vi "Live Capture Functional Stack.12.64bit.vi"() -> ()   [LabVIEW 2014]
uses:
  subvis/Stack Track.ctl
  subvis/Stack_State.ctl
  CameraControlTypeDef.ctl
  Desktop/camtiff/ctiff.llb/__CTIFFNewFileAndStyleUINT16.vi
  Desktop/camtiff/ctiff.llb/__CTIFFAddNewPageUINT16.vi
panel:
  out "Stacks":i32
  in  "ROI":bool
  out "Video":T1(plugin-control)
  out "Internal Line Interval":dbl
  in  "Mode":bool
  in  "Preview":bool
  in  "Capture Mode":bool
  out "Record Ready":bool
  in  "Stacks":dbl=1.0
  out "Stack Frames":i32=100
  in  "Stack Frames":i32=100
  in  "Temp":path=path "C:/temp.tmp"
  in  "Frames":i32=100
  in  "HardDisk Record":bool
  in  "Internal Line Interval":dbl
  in  "Slit Width / Lines":sgl=150.0
  in  "Camera Readout Mode":u16(ring)=12 items=["Full Frame"=1, "Slit Scanning"=12]
  in  "Readout Direction":sgl(ring)=1.0 items=["Forward"=1, "Backward"=2]
  in  "Trigger Mode":sgl(ring)=1.0 items=["Normal"=1, "Start "=6]
  in  "Trigger Source":sgl(ring)=2.0 items=["Internal"=1, "External"=2]
  out "State":T2=enum."Start Sequence"
  out "Saving":bool
  in  "AutoIncrement":bool=TRUE
  in  "Path":path=path "C:/Users/spim/Desktop/Craig Cap/temp/a.tiff"
  in  "Frames":i32=100
  out "Frame Index":i32
  out "error out":errorcluster
  in  "stop":bool
  in  "Ram Record":bool
  out "Total Frames":i32
  out "Elapsed Time":u32
  out "Software FPS":dbl
  out "Camera FPS":dbl
  in  "H Offset":i32 min=0 max=0 step=4
  in  "H Width":i32 min=4 max=2048 step=4
  out "SMD":dbl
  out "SHO":i32
  in  "V Offset":i32 min=0 max=0 step=4
  in  "V Width":i32 min=4 max=2048 step=4
  in  "Binning":u16(ring) items=["1x1"=1, "2x2"=2, "4x4"=4]
  out "SHW":i32
  out "SVO":i32
  out "SVW":i32
  in  "Scan Mode":dbl min=1.0 max=2.0 step=1.0
  in  "Exposure":dbl min=0.0010036691729323308 max=10.000004210526315 step=1e-08
  out "EXP":dbl
  out "Camera Model":string
  out "Camera Version":string
  out "Camera Serial":string
  # "Broked"
  # "XYT \nXYZ\nXYTZ\nXYZT"
  # "Capture Mode"
  # "Preview Mode"
  # "HDD superior, will not drop frames or stacks"
  # "Change to rock switch"
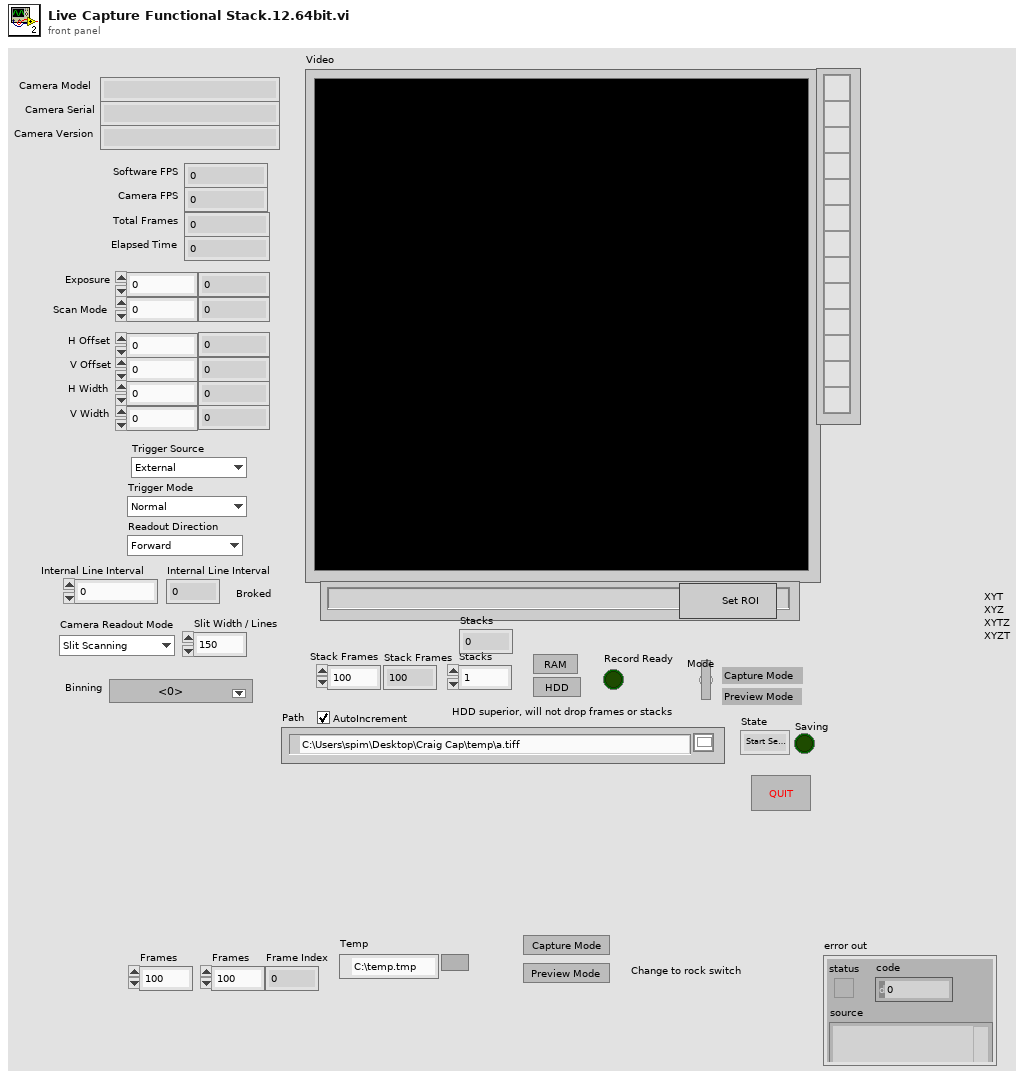
[diagram p1: front panel]
types:
  T1 = typedef "IMAQ Image.ctl" = refnum<image>
  T2 = typedef "Stack Track.ctl" = enum16{"Idle", "Start Sequence", "Read Disk", "STOP", "Collecting", "End"}
  T3 = typedef "CameraControlTypeDef.ctl" = enum16{"IntervalLineInt", "Ram Record", "HardDisk Record", "Disengage Update", "Update", "Idle", "ROI", "Binning", "Scan Mode", "Trigger Mode", "Readout Mode", "Readout Direction", "Preview", "ROIWindow", "Trigger Source"}
  T4 = typedef "Stack_State.ctl" = cluster{"State":T2, "Stack Number":i32, "Image":u16[][], "Stacks":i32}
  T5 = enum8{"Enabled", "Disabled", "Disabled and Grayed Out"}
  T6 = typedef "Image Type" = u32
  T7 = cluster{"Model":string, "Camera ID":string, "Firmware":string}
  T8 = cluster{"Value":i32, "Minimum":i32, "Maximum":i32, "Increment":i32}
  T9 = cluster{"height":u32, "width":u32, "datatype":u32}
  T10 = cluster{"H Offset":i32, "V Offset":i32, "H Width":i32, "V Width":i32}
  T11 = typedef "ROI Descriptor" = cluster{"Global Rectangle":i32[], "Contours":cluster{"ID":enum32{"External", "Internal"}, "Type":u32, "Coordinates":i32[]}[]}
  T12 = cluster{"ID":enum32{"External", "Internal"}, "Type":u32, "Coordinates":i32[]}[]
  T13 = cluster{"ID":enum32{"External", "Internal"}, "Type":u32, "Coordinates":i32[]}
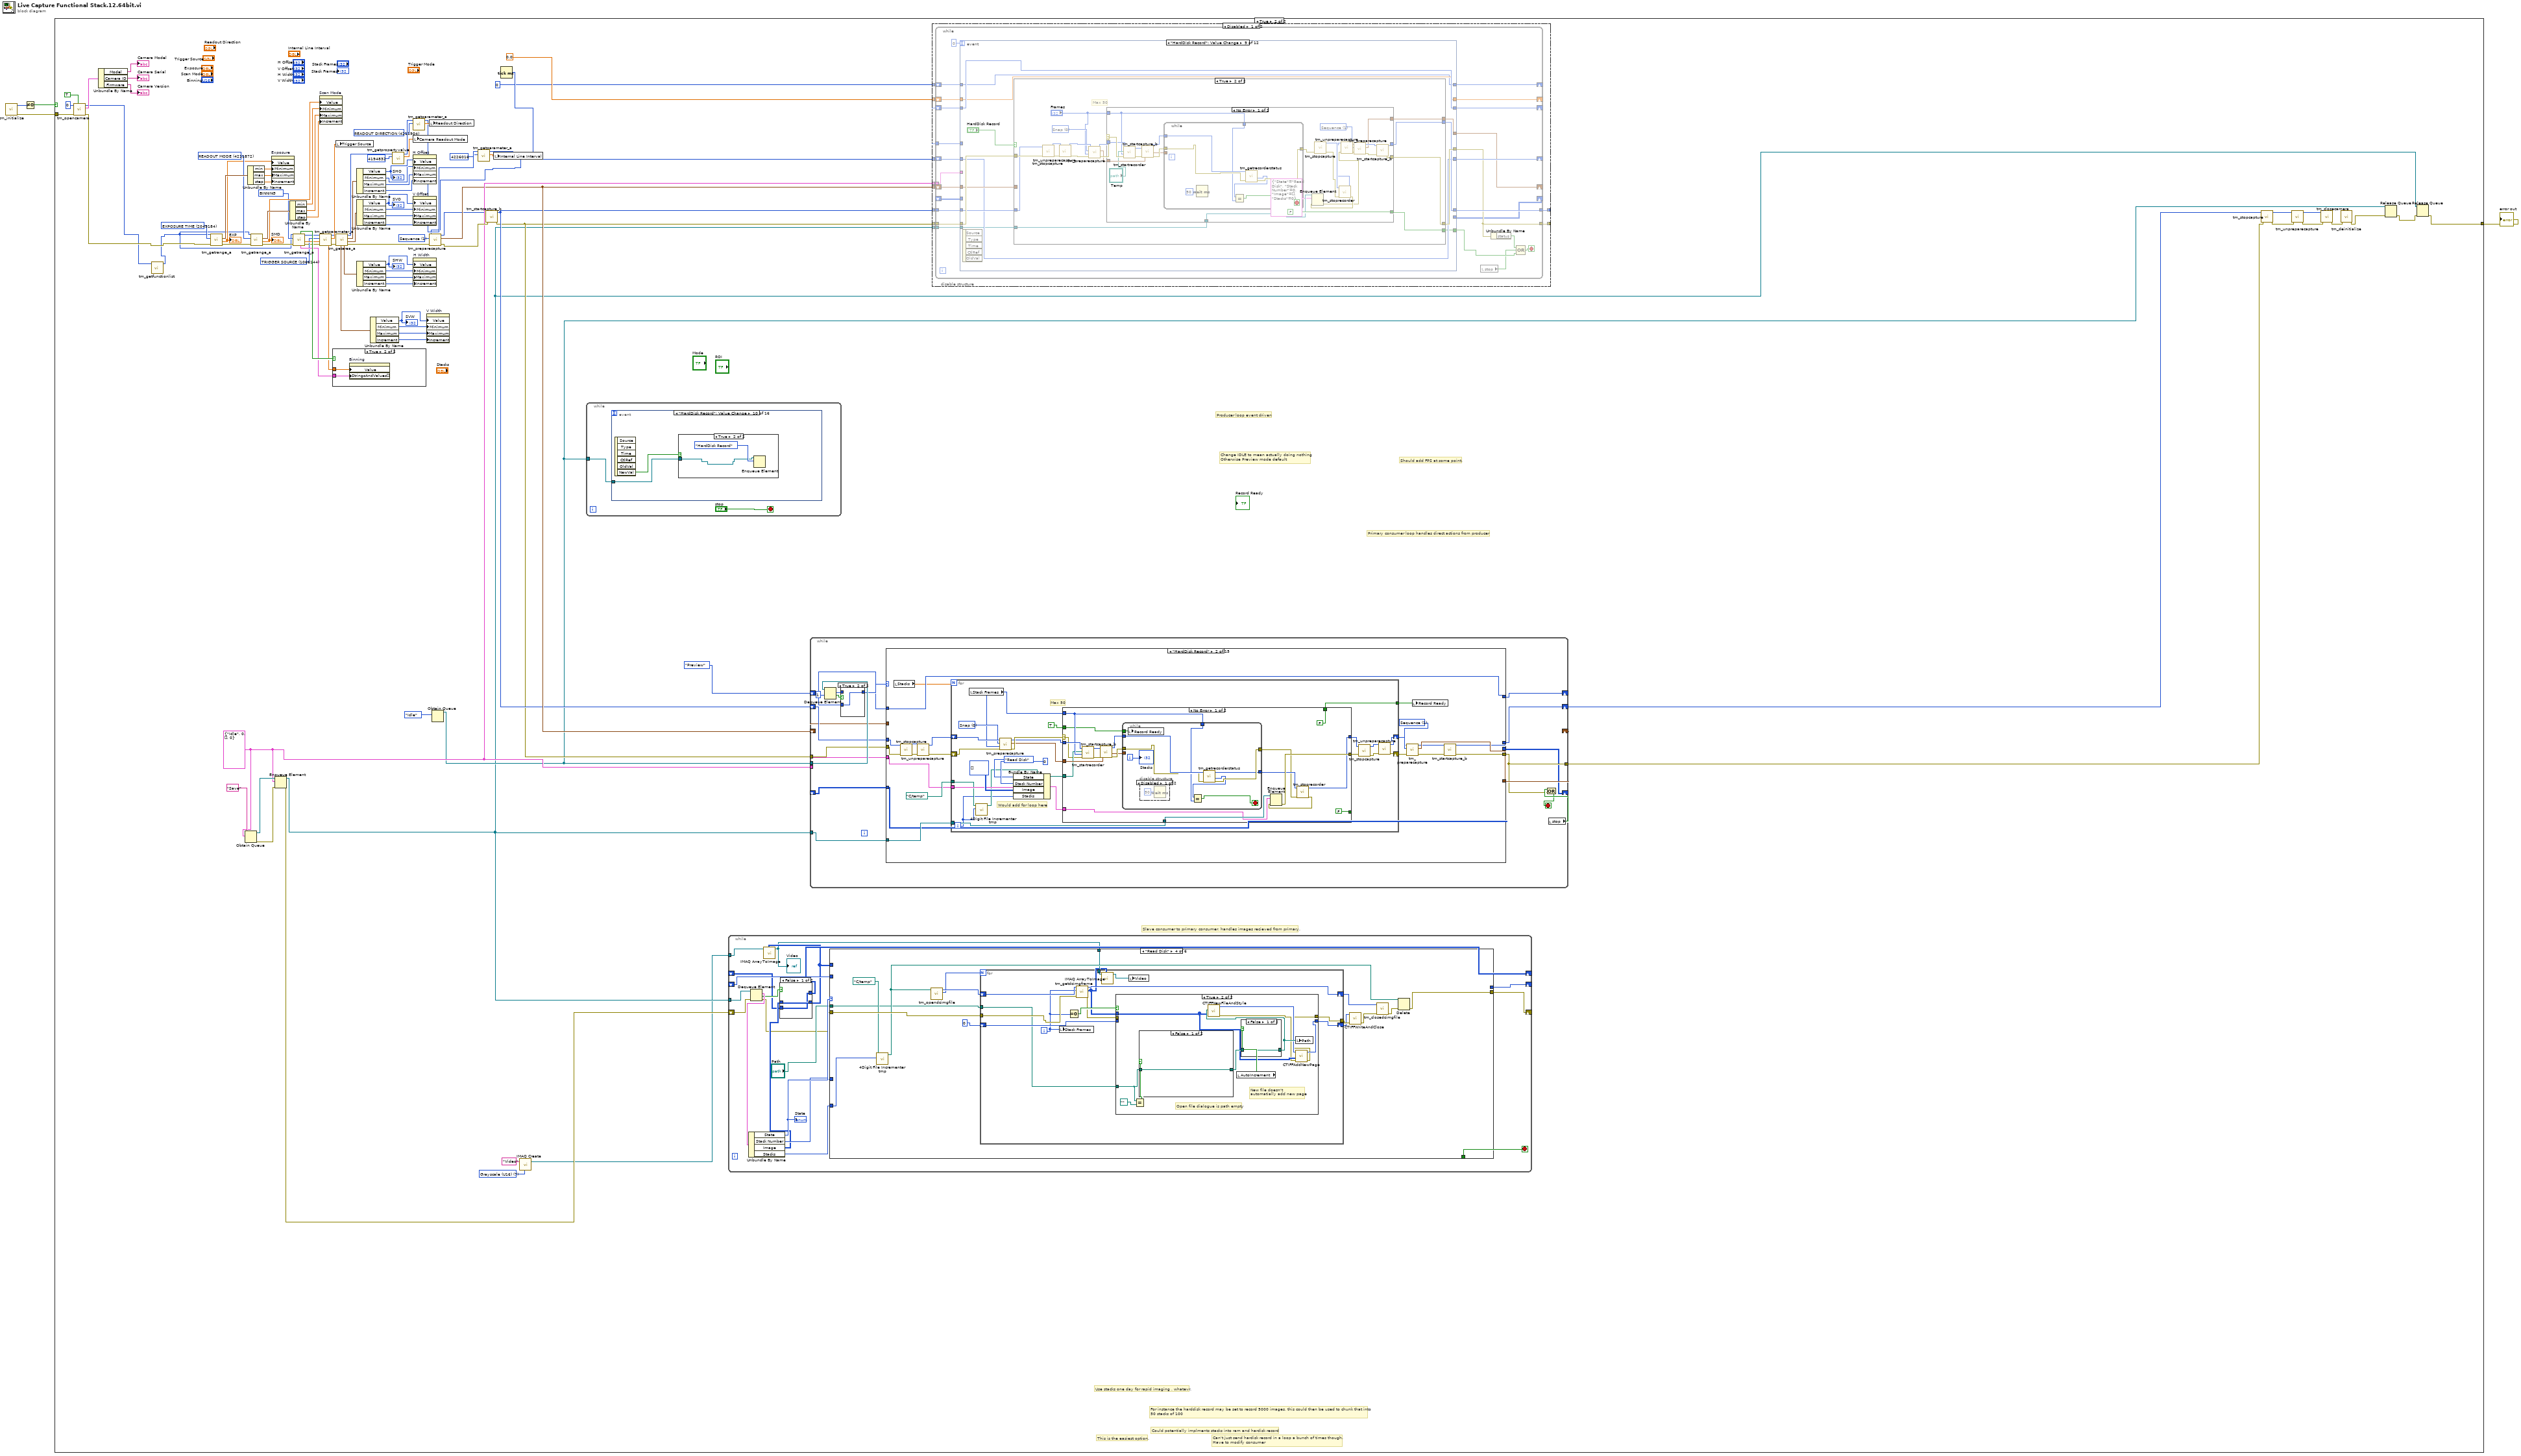
[diagram p0: block diagram]
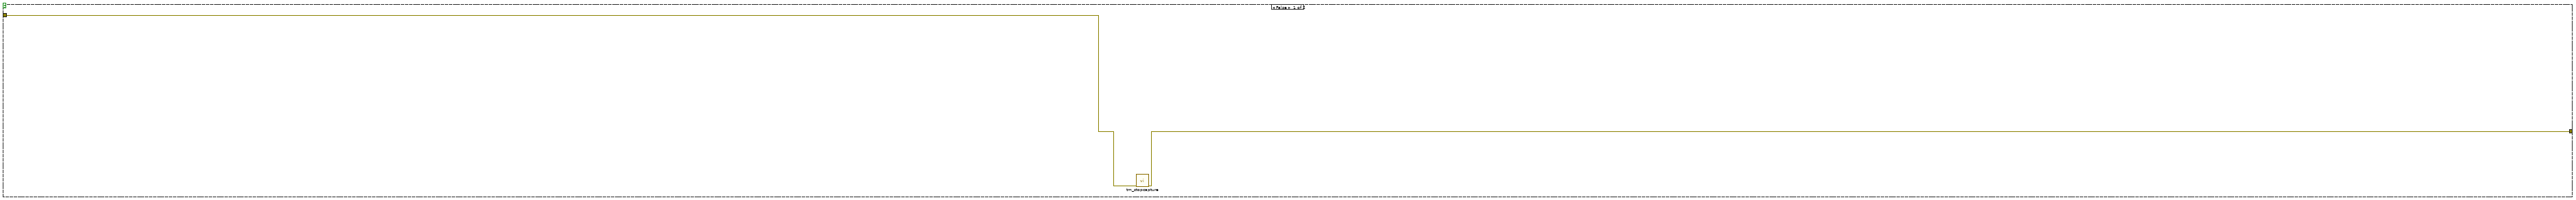
[diagram p2: hidden frame]
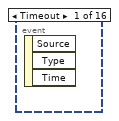
[diagram p3: hidden frame]
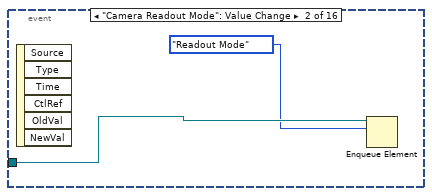
[diagram p4: hidden frame]
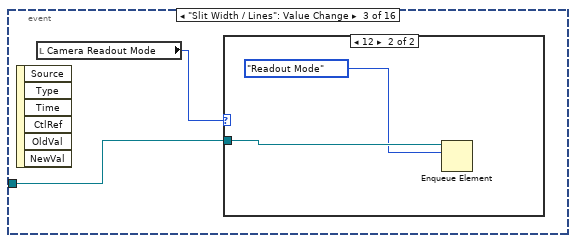
[diagram p5: hidden frame]
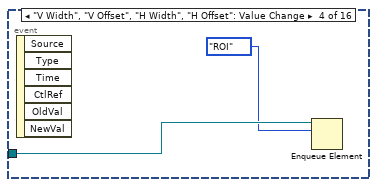
[diagram p7: hidden frame]
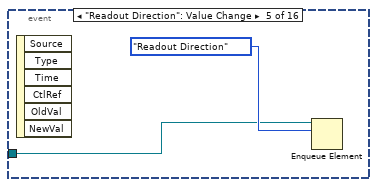
[diagram p8: hidden frame]
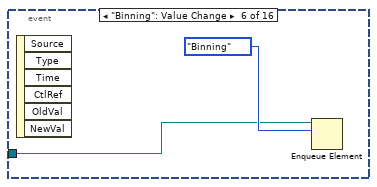
[diagram p9: hidden frame]
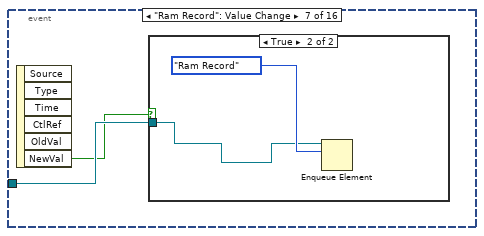
[diagram p10: hidden frame]
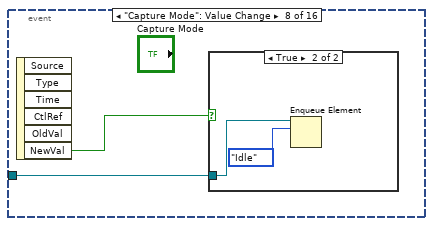
[diagram p12: hidden frame]
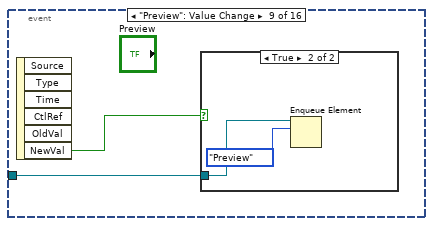
[diagram p14: hidden frame]
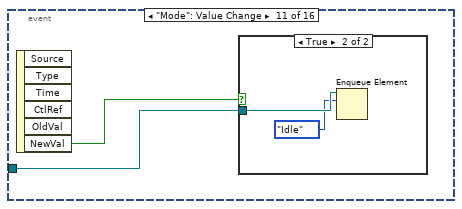
[diagram p17: hidden frame]
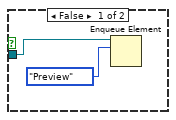
[diagram p18: hidden frame]
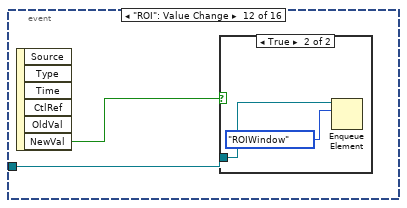
[diagram p19: hidden frame]
diagram:
  n1 = call <userlib>:"tm_initialize.vi"() -> ("error out"=w2:errorcluster, "Number Of Cameras"=w1:u32)  [unwired: 8 in, 2 out]
  n2 = Not Equal To 0?(x=w1) -> (x != 0?=w4:bool)
  n3 = case shown="True" w4 {
    tunnel: [w5 w19] -> w3
    tunnel: w2 -> [w6 w102]
    frame False {
      n4 = call <userlib>:"tm_stopcapture.vi"("error in (no error)"=w6) -> ("error out"=w5:errorcluster)  [unwired: 9 in, 1 out]
    }
    frame True {
      w9 = T6 7 items=["Grayscale (U8)", "Grayscale (I16)", "Grayscale (SGL)", "Complex (CSG)", "RGB (U32)", "HSL (U32)", "RGB (U64)", "Grayscale (U16)"] ("Image Type")
      w37 = u32 4211904 items=["SENSOR MODE"=4212128, "CCD MODE"=4212384, "READOUT MODE"=4211872, "ACTIVE VIEW INDEX"=4343136, "BITS PER CHANNEL"=4342976, "IMAGE PIXEL TYPE"=4343296, "BINNING"=4215968, "EXPOSURE TIME"=2049184, "CONTRAST GAIN"=3163312, "CONTRAST OFFSET"=3163328, "LIGHT MODE"=2114720, "SENSITIVITY"=2114992, "PHOTON IMAGING MODE"=2115200, "HIGH DYNAMIC RANGE MODE"=3163360, "WHITE BALANCE"=3163568, "TEMPERATURE"=2115232, "TEMPERATURE TARGET"=2115264, "SENSOR COOLER FAN"=2115296, "LINEBUNDLE HEIGHT"=4212192, "MECHANICAL SHUTTER"=2115488, "BACK FOCUS POSITION"=8422304, "TRIGGER CONNECTOR"=1066432, "TRIGGER SOURCE"=1066144, "OUTPUT TRIGGER SOURCE"=1852576, "TRIGGER GLOBAL EXPOSURE"=2049680, "FIRST TRIGGER BEHAVIOR"=2049696, "CHANNEL SYNC"=1852352, "READOUT DIRECTION"=4211904, "PRE HSYNC COUNT"=1852704] ("Parameter")
      w46 = u32 1066144 items=["SENSOR MODE"=4212128, "CCD MODE"=4212384, "READOUT MODE"=4211872, "ACTIVE VIEW INDEX"=4343136, "BITS PER CHANNEL"=4342976, "IMAGE PIXEL TYPE"=4343296, "BINNING"=4215968, "EXPOSURE TIME"=2049184, "CONTRAST GAIN"=3163312, "CONTRAST OFFSET"=3163328, "LIGHT MODE"=2114720, "SENSITIVITY"=2114992, "PHOTON IMAGING MODE"=2115200, "HIGH DYNAMIC RANGE MODE"=3163360, "WHITE BALANCE"=3163568, "TEMPERATURE"=2115232, "TEMPERATURE TARGET"=2115264, "SENSOR COOLER FAN"=2115296, "LINEBUNDLE HEIGHT"=4212192, "MECHANICAL SHUTTER"=2115488, "BACK FOCUS POSITION"=8422304, "TRIGGER CONNECTOR"=1066432, "TRIGGER SOURCE"=1066144, "OUTPUT TRIGGER SOURCE"=1852576, "TRIGGER GLOBAL EXPOSURE"=2049680, "FIRST TRIGGER BEHAVIOR"=2049696, "CHANNEL SYNC"=1852352, "READOUT DIRECTION"=4211904, "PRE HSYNC COUNT"=1852704] ("Parameter")
      w32 = T4 {"State"=enum."Idle", "Stack Number"=0, "Image"=[], "Stacks"=0} ("input cluster")
      w51 = u32 2049184 items=["BINNING"=4215968, "BITS PER CHANNEL"=4342976, "ACTIVE VIEW INDEX"=4343136, "CCD MODE"=4212384, "SENSOR MODE"=4212128, "READOUT MODE"=4211872, "EXPOSURE TIME"=2049184, "CONTRAST GAIN"=3163312, "CONTRAST OFFSET"=3163328, "LIGHT MODE"=2114720, "SENSITIVITY"=2114992, "WHITE BALANCE"=3163568, "PHOTON IMAGING MODE"=2115200, "HIGH DYNAMIC RANGE MODE"=3163360, "TRIGGER SOURCE"=1066144, "TRIGGER ACTIVE"=1066160, "TRIGGER MODE"=1066400, "TRIGGER POLARITY"=1066416, "TRIGGER GLOBAL EXPOSURE"=2049680, "FIRST TRIGGER BEHAVIOR"=2049696, "TRIGGER TIMES"=1066448, "OUTPUT TRIGGER POLARITY"=1852592, "OUTPUT TRIGGER DELAY"=1852624, "OUTPUT TRIGGER PERIOD"=1852640, "TEMPERATURE"=2115232, "TEMPERATURE TARGET"=2115264, "SENSOR COOLER FAN"=2115296, "MECHANICAL SHUTTER"=2115488, "BACK FOCUS POSITION"=8422304, "FRAMEBUNDLE MODE"=4346784, "FRAMEBUNDLE NUMBER"=4346800, "LINEBUNDLE HEIGHT"=4212192, "TRIGGER CONNECTOR"=1066432, "IMAGE PIXEL TYPE"=4343296, "OUTPUT TRIGGER KIND"=1852656, "READOUT DIRECTION"=4211904, "CHANNEL SYNC"=1852352] ("Parameter")
      w52 = u32 4211872 items=["BINNING"=4215968, "BITS PER CHANNEL"=4342976, "ACTIVE VIEW INDEX"=4343136, "CCD MODE"=4212384, "SENSOR MODE"=4212128, "READOUT MODE"=4211872, "EXPOSURE TIME"=2049184, "CONTRAST GAIN"=3163312, "CONTRAST OFFSET"=3163328, "LIGHT MODE"=2114720, "SENSITIVITY"=2114992, "WHITE BALANCE"=3163568, "PHOTON IMAGING MODE"=2115200, "HIGH DYNAMIC RANGE MODE"=3163360, "TRIGGER SOURCE"=1066144, "TRIGGER ACTIVE"=1066160, "TRIGGER MODE"=1066400, "TRIGGER POLARITY"=1066416, "TRIGGER GLOBAL EXPOSURE"=2049680, "FIRST TRIGGER BEHAVIOR"=2049696, "TRIGGER TIMES"=1066448, "OUTPUT TRIGGER POLARITY"=1852592, "OUTPUT TRIGGER DELAY"=1852624, "OUTPUT TRIGGER PERIOD"=1852640, "TEMPERATURE"=2115232, "TEMPERATURE TARGET"=2115264, "SENSOR COOLER FAN"=2115296, "MECHANICAL SHUTTER"=2115488, "BACK FOCUS POSITION"=8422304, "FRAMEBUNDLE MODE"=4346784, "FRAMEBUNDLE NUMBER"=4346800, "LINEBUNDLE HEIGHT"=4212192, "TRIGGER CONNECTOR"=1066432, "IMAGE PIXEL TYPE"=4343296, "OUTPUT TRIGGER KIND"=1852656, "READOUT DIRECTION"=4211904, "CHANNEL SYNC"=1852352] ("Parameter")
      w53 = u32 4215968 items=["BINNING"=4215968, "BITS PER CHANNEL"=4342976, "ACTIVE VIEW INDEX"=4343136, "CCD MODE"=4212384, "SENSOR MODE"=4212128, "READOUT MODE"=4211872, "EXPOSURE TIME"=2049184, "CONTRAST GAIN"=3163312, "CONTRAST OFFSET"=3163328, "LIGHT MODE"=2114720, "SENSITIVITY"=2114992, "WHITE BALANCE"=3163568, "PHOTON IMAGING MODE"=2115200, "HIGH DYNAMIC RANGE MODE"=3163360, "TRIGGER SOURCE"=1066144, "TRIGGER ACTIVE"=1066160, "TRIGGER MODE"=1066400, "TRIGGER POLARITY"=1066416, "TRIGGER GLOBAL EXPOSURE"=2049680, "FIRST TRIGGER BEHAVIOR"=2049696, "TRIGGER TIMES"=1066448, "OUTPUT TRIGGER POLARITY"=1852592, "OUTPUT TRIGGER DELAY"=1852624, "OUTPUT TRIGGER PERIOD"=1852640, "TEMPERATURE"=2115232, "TEMPERATURE TARGET"=2115264, "SENSOR COOLER FAN"=2115296, "MECHANICAL SHUTTER"=2115488, "BACK FOCUS POSITION"=8422304, "FRAMEBUNDLE MODE"=4346784, "FRAMEBUNDLE NUMBER"=4346800, "LINEBUNDLE HEIGHT"=4212192, "TRIGGER CONNECTOR"=1066432, "IMAGE PIXEL TYPE"=4343296, "OUTPUT TRIGGER KIND"=1852656, "READOUT DIRECTION"=4211904, "CHANNEL SYNC"=1852352] ("Parameter")
      w98 = 1 items=["Snap", "Sequence"] ("Capture mode")
      # "Slave consumer to primary consumer, handles images recieved from primary."
      # "Can't just send hardisk record in a loop a bunch of times though.\nHave to modify consumer"
      # "This is the easiest option."
      # "Could potentially implments stacks into ram and hardisk record"
      # "For instance the harddisk record may be set to record 5000 images, this could then be used to chunk that into\n50 stacks of 100"
      # "Use stacks one day for rapid imaging , whatevr."
      # "Change IDLE to mean actually doing nothing\nOtherwise Preview mode default"
      # "Primary consumer loop handles direct actions from producer"
      # "Producer loop event driven"
      # "Should add FPS at some point."
      n5 = call <userlib>:"tm_opencamera.vi"("Force Open"=TRUE, "error in (no error)"=w102, "Camera Index"=u32 0) -> ("error out"=w33:errorcluster, "Camera Details"=w65:T7, "Handle out"=w17:u32)  [unwired: 6 in]
      n6 = Unbundle By Name(w65) -> ("Model"=→"Camera Model":string, "Camera ID"=→"Camera Serial":string, "Firmware"=→"Camera Version":string)
      n7 = call <userlib>:"tm_getfunctionlist.vi"("Handle in"=w17) -> ("Handle out"=w16:u32)  [unwired: 8 in, 2 out]
      n8 = call <userlib>:"tm_getrange_a.vi"("error in (no error)"=w33, "Parameter"=w51, "Handle in"=w16) -> ("error out"=w60:errorcluster, "default"=w49:dbl, "Range"=w61:cluster{"min":dbl, "max":dbl, "step":dbl})  [unwired: 2 in, 4 out]
      "EXP" <- w49
      n9 = Obtain Queue(name (unnamed)="Save", element data type=w32) -> (queue out=w35:refnum<queue>, error out=w14:errorcluster)  [unwired: 3 in, 1 out]
      n10 = Unbundle By Name(w61) -> ("min"=w96:dbl, "max"=w95:dbl, "step"=w94:dbl)
      n11 = call <userlib>:"tm_getrange_a.vi"("error in (no error)"=w60, "Parameter"=w52, "Handle in"=w16) -> ("error out"=w57:errorcluster, "default"=w58:dbl, "Range"=w59:cluster{"min":dbl, "max":dbl, "step":dbl})  [unwired: 2 in, 4 out]
      "SMD" <- w58
      n12 = property on="Exposure" class="DigNum (strict)"("Value"=w49, "Minimum"=w96, "Maximum"=w95, "Increment"=w94) -> ()  [unwired: 2 in, 2 out]
      n13 = Enqueue Element(queue=w35, element=w32, error in (no error)=w14) -> (queue out=w18:refnum<queue>, error out=w13:errorcluster)  [unwired: 1 in, 1 out]
      n14 = Unbundle By Name(w59) -> ("min"=w93:dbl, "max"=w92:dbl, "step"=w91:dbl)
      n15 = call <userlib>:"tm_getrange_a.vi"("error in (no error)"=w57, "Parameter"=w53, "Handle in"=w16) -> ("error out"=w43:errorcluster, "default"=w55:dbl, "Handle out"=w45:u32, "Value Names"=w54:cluster{"Name":string, "Value":dbl}[], "Writable"=w56:bool)  [unwired: 2 in, 2 out]
      n16 = property on="Scan Mode" class="DigNum (strict)"("Value"=w58, "Minimum"=w93, "Maximum"=w92, "Increment"=w91) -> ()  [unwired: 2 in, 2 out]
      n17 = call <userlib>:"tm_getparameter_a.vi"("error in (no error)"=w43, "Parameter"=w46, "Handle in"=w45) -> ("error out"=w42:errorcluster, "Value out"=w47:dbl, "Handle out"=w44:u32)  [unwired: 6 in]
      n18 = case shown="True" w56 {
        tunnel: w54 -> [_ w1289]
        tunnel: w55 -> [_ w1288]
        frame False {
        }
        frame True {
          n19 = property on="Binning" class="Ring (strict)"("Value"=w1288, "StringsAndValues[]"=w1289) -> ()  [unwired: 2 in, 2 out]
        }
      }
      n20 = local write "Trigger Source"(w47) -> ()
      n21 = call <userlib>:"tm_getarea_a.vi"("error in (no error)"=w42, "Handle in"=w44) -> ("error out"=w48:errorcluster, "V Offset"=w90:T8, "H Offset"=w71:T8, "Handle out"=w39:u32, "H Width"=w89:T8, "V Width"=w88:T8)  [unwired: 4 in]
      n22 = Unbundle By Name(w71) -> ("Value"=w70:i32, "Minimum"=w69:i32, "Maximum"=w68:i32, "Increment"=w67:i32)
      "SHO" <- w70
      n23 = Unbundle By Name(w90) -> ("Value"=w78:i32, "Minimum"=w87:i32, "Maximum"=w86:i32, "Increment"=w85:i32)
      "SVO" <- w78
      n24 = Unbundle By Name(w89) -> ("Value"=w77:i32, "Minimum"=w84:i32, "Maximum"=w83:i32, "Increment"=w82:i32)
      "SHW" <- w77
      n25 = Unbundle By Name(w88) -> ("Value"=w76:i32, "Minimum"=w81:i32, "Maximum"=w80:i32, "Increment"=w79:i32)
      "SVW" <- w76
      n26 = call <userlib>:"tm_getpropertyvalue.vi"("Property ID"=u32 4194832, "Handle in"=w39) -> ("Value in"=w40:sgl, "Handle out"=w38:u32)  [unwired: 7 in, 1 out]
      n27 = call <userlib>:"tm_getparameter_a.vi"("Parameter"=w37, "Handle in"=w38) -> ("Value out"=w36:dbl, "Handle out"=w23:u32)  [unwired: 7 in, 1 out]
      n28 = local write "Camera Readout Mode"(w40) -> ()
      n29 = property on="H Offset" class="DigNum (strict)"("Value"=w70, "Minimum"=w69, "Maximum"=w68, "Increment"=w67) -> ()  [unwired: 2 in, 2 out]
      n30 = property on="V Offset" class="DigNum (strict)"("Value"=w78, "Minimum"=w87, "Maximum"=w86, "Increment"=w85) -> ()  [unwired: 2 in, 2 out]
      n31 = property on="H Width" class="DigNum (strict)"("Value"=w77, "Minimum"=w84, "Maximum"=w83, "Increment"=w82) -> ()  [unwired: 2 in, 2 out]
      n32 = property on="V Width" class="DigNum (strict)"("Value"=w76, "Minimum"=w81, "Maximum"=w80, "Increment"=w79) -> ()  [unwired: 2 in, 2 out]
      n33 = local write "Readout Direction"(w36) -> ()
      n34 = Obtain Queue(element data type=CameraControlTypeDef."Idle" ("Enum")) -> (queue out=w21:refnum<queue>)  [unwired: 4 in, 2 out]
      n35 = call <userlib>:"tm_getparameter_a.vi"("Parameter"=4226016, "Handle in"=w23) -> ("Value out"=w11:dbl, "Handle out"=w12:u32)  [unwired: 7 in, 1 out]
      n36 = call <userlib>:"tm_preparecapture.vi"("error in (no error)"=w48, "Capture mode"=w98, "Handle in"=w12) -> ("error out"=w34:errorcluster, "Buffer Info"=w31:T9, "Handle out"=w24:u32)  [unwired: 5 in, 1 out]
      n37 = call <userlib>:"tm_startcapture_b.vi"("error in (no error)"=w34, "Handle in"=w24) -> ("error out"=w29:errorcluster, "Handle out"=w30:u32)  [unwired: 8 in]
      n38 = local write "Internal Line Interval"(w11) -> ()
      n39 = Tick Count (ms)() -> (millisecond timer value=w97:u32)
      n40 = call "IMAQ Create"("Image Name"="Video", "Image Type"=w9) -> ("New Image"=w8:T1)  [unwired: 3 in, 1 out]
      n41 = while {
        tunnel: w21 -> [w104]
        stop <- "stop" stop-if-true
        n42 = event shown="[9] \"HardDisk Record\": Value Change" {
          selector: _ -> [_ _ _ _ _ _ _ _ _ _ _ _ _ _ _ _]
          dyn-events: _ -> [_ _ _ _ _ _ _ _ _ _ _ _ _ _ _ _]
          timeout: _ -> [_ _ _ _ _ _ _ _ _ _ _ _ _ _ _ _]
          tunnel: w104 -> [_ w106 w108 w112 w113 w115 w118 w121 w125 w130 w133 w139 w143 w147 w159 w171]
          event Timeout {
            n43 = event-data() -> ()  [unwired: 1 in, 3 out]
          }
          event "Camera Readout Mode": Value Change {
            n44 = event-data() -> ()  [unwired: 1 in, 6 out]
            n45 = Enqueue Element(queue=w106, element=CameraControlTypeDef."Readout Mode" ("Enum")) -> ()  [unwired: 2 in, 3 out]
          }
          event "Slit Width / Lines": Value Change {
            n46 = event-data() -> ()  [unwired: 1 in, 6 out]
            n47 = local read "Camera Readout Mode"() -> (w107:u16)
            n48 = case shown="12" w107 {
              tunnel: w108 -> [_ w110]
              frame 0, Default {
              }
              frame 12 {
                n49 = Enqueue Element(queue=w110, element=CameraControlTypeDef."Readout Mode" ("Enum")) -> ()  [unwired: 2 in, 3 out]
              }
            }
          }
          event "V Width", "V Offset", "H Width", "H Offset": Value Change {
            n50 = event-data() -> ()  [unwired: 1 in, 6 out]
            n51 = Enqueue Element(queue=w112, element=CameraControlTypeDef."ROI" ("Enum")) -> ()  [unwired: 2 in, 3 out]
          }
          event "Readout Direction": Value Change {
            n52 = event-data() -> ()  [unwired: 1 in, 6 out]
            n53 = Enqueue Element(queue=w113, element=CameraControlTypeDef."Readout Direction" ("Enum")) -> ()  [unwired: 2 in, 3 out]
          }
          event "Binning": Value Change {
            n54 = event-data() -> ()  [unwired: 1 in, 6 out]
            n55 = Enqueue Element(queue=w115, element=CameraControlTypeDef."Binning" ("Enum")) -> ()  [unwired: 2 in, 3 out]
          }
          event "Ram Record": Value Change {
            n56 = event-data() -> ("NewVal"=w117:bool)  [unwired: 1 in, 5 out]
            n57 = case shown="True" w117 {
              tunnel: w118 -> [_ w119]
              frame False {
              }
              frame True {
                n58 = Enqueue Element(queue=w119, element=CameraControlTypeDef."Ram Record" ("Enum")) -> ()  [unwired: 2 in, 3 out]
              }
            }
          }
          event "Capture Mode": Value Change {
            n59 = event-data() -> ("NewVal"=w122:bool)  [unwired: 1 in, 5 out]
            n60 = case shown="True" w122 {
              tunnel: w121 -> [_ w124]
              frame False {
              }
              frame True {
                n61 = Enqueue Element(queue=w124, element=CameraControlTypeDef."Idle") -> ()  [unwired: 2 in, 3 out]
              }
            }
          }
          event "Preview": Value Change {
            n62 = event-data() -> ("NewVal"=w126:bool)  [unwired: 1 in, 5 out]
            n63 = case shown="True" w126 {
              tunnel: w125 -> [_ w128]
              frame False {
              }
              frame True {
                n64 = Enqueue Element(queue=w128, element=CameraControlTypeDef."Preview") -> ()  [unwired: 2 in, 3 out]
              }
            }
          }
          event "HardDisk Record": Value Change {
            n65 = event-data() -> ("NewVal"=w129:bool)  [unwired: 1 in, 5 out]
            n66 = case shown="True" w129 {
              tunnel: w130 -> [_ w131]
              frame False {
              }
              frame True {
                n67 = Enqueue Element(queue=w131, element=CameraControlTypeDef."HardDisk Record" ("Enum")) -> ()  [unwired: 2 in, 3 out]
              }
            }
          }
          event "Mode": Value Change {
            n68 = event-data() -> ("NewVal"=w134:bool)  [unwired: 1 in, 5 out]
            n69 = case shown="True" w134 {
              tunnel: w133 -> [w135 w138]
              frame False {
                n70 = Enqueue Element(queue=w135, element=CameraControlTypeDef."Preview") -> ()  [unwired: 2 in, 3 out]
              }
              frame True {
                n71 = Enqueue Element(queue=w138, element=CameraControlTypeDef."Idle") -> ()  [unwired: 2 in, 3 out]
              }
            }
          }
          event "ROI": Value Change {
            n72 = event-data() -> ("NewVal"=w140:bool)  [unwired: 1 in, 5 out]
            n73 = case shown="True" w140 {
              tunnel: w139 -> [_ w141]
              frame False {
              }
              frame True {
                n74 = Enqueue Element(queue=w141, element=CameraControlTypeDef."ROIWindow") -> ()  [unwired: 2 in, 3 out]
              }
            }
          }
          event "Exposure": Value Change {
            n75 = event-data() -> ()  [unwired: 1 in, 6 out]
            n76 = Enqueue Element(queue=w143, element=CameraControlTypeDef."Update" ("Enum")) -> ()  [unwired: 2 in, 3 out]
          }
          event "Trigger Source": Value Change {
            n77 = event-data() -> ("NewVal"=w145:sgl)  [unwired: 1 in, 5 out]
            n78 = case shown="2" w145 {
              tunnel: w147 -> [w151 w155]
              tunnel: [w150 w154] -> w146
              frame 2 {
                n79 = local write "Mode"(TRUE ("Mode")) -> ()
                n80 = Enqueue Element(queue=w151, element=CameraControlTypeDef."Idle" ("Enum")) -> (queue out=w150:refnum<queue>)  [unwired: 2 in, 2 out]
              }
              frame 1, Default {
                n81 = local write "Mode"(FALSE ("Mode")) -> ()
                n82 = Enqueue Element(queue=w155, element=CameraControlTypeDef."Preview" ("Enum")) -> (queue out=w154:refnum<queue>)  [unwired: 2 in, 2 out]
              }
            }
            n83 = Enqueue Element(queue=w146, element=CameraControlTypeDef."Trigger Source" ("Enum")) -> ()  [unwired: 2 in, 3 out]
          }
          event "Trigger Mode": Value Change {
            n84 = event-data() -> ("NewVal"=w157:sgl)  [unwired: 1 in, 5 out]
            n85 = case shown="6" w157 {
              tunnel: w159 -> [w163 w167]
              tunnel: [w162 w166] -> w158
              frame 6 {
                n86 = local write "Mode"(TRUE ("Mode")) -> ()
                n87 = Enqueue Element(queue=w163, element=CameraControlTypeDef."Idle" ("Enum")) -> (queue out=w162:refnum<queue>)  [unwired: 2 in, 2 out]
              }
              frame 1, Default {
                n88 = local write "Mode"(FALSE ("Mode")) -> ()
                n89 = Enqueue Element(queue=w167, element=CameraControlTypeDef."Preview" ("Enum")) -> (queue out=w166:refnum<queue>)  [unwired: 2 in, 2 out]
              }
            }
            n90 = Enqueue Element(queue=w158, element=CameraControlTypeDef."Trigger Mode" ("Enum")) -> ()  [unwired: 2 in, 3 out]
          }
          event "Internal Line Interval": Value Change {
            n91 = event-data() -> ("OldVal"=w170:dbl)  [unwired: 1 in, 5 out]
            n92 = Enqueue Element(queue=w171, element=CameraControlTypeDef."IntervalLineInt", timeout in ms (-1)=w170) -> ()  [unwired: 1 in, 3 out]
          }
        }
      }
      n93 = while {
        tunnel: w18 -> [w1200]
        shift-right: [w1196] -> _
        shift-left: _ -> [w1194]
        shift-right: [w1193] -> _
        shift-left: w13 -> [w1187]
        shift-right: [w1191] -> _
        shift-left: _ -> [w1188]
        tunnel: w8 -> [w1184]
        stop <- w1195 stop-if-true
        n94 = Dequeue Element(queue=w1200, error in (no error)=w1187) -> (element=w1199:T4, timed out?=w1189:bool, error out=w1186:errorcluster)  [unwired: 1 in, 1 out]
        n95 = Unbundle By Name(w1199) -> ("State"=w1198:T2, "Stack Number"=w1197:i32, "Image"=w1190:u16[][], "Stacks"=w1185:i32)
        "State" <- w1198
        n96 = case shown="False" w1189 {
          tunnel: w1190 -> [w1202 w1204]
          tunnel: [w1202 w1203] -> w1183
          tunnel: [w1201 w1204] -> w1191
          tunnel: w1188 -> [w1201 w1203]
          frame False {
          }
          frame True {
          }
        }
        n97 = call "IMAQ ArrayToImage"("Image Pixels (U16)"=w1183, "Image"=w1184) -> ("Image Out"=w1182:T1)  [unwired: 8 in, 1 out]
        "Video" <- w1182
        n98 = case shown="\"Read Disk\"" w1198 {
          tunnel: w1197 -> [_ _ _ _ _ _]
          tunnel: [w1207 w1224 _ _ _ _] -> w1196
          tunnel: w1194 -> [_ w1225 w1231 _ _ _]
          tunnel: [FALSE _ _ _ TRUE _] -> w1195
          tunnel: w1183 -> [w1205 w1226 _ _ _ _]
          tunnel: w1186 -> [_ w1223 w1229 w1245 w1285 w1287]
          tunnel: [w1208 w1222 w1230 w1242 w1285 w1287] -> w1193
          tunnel: "Path" -> [w1211 _ _ w1235 _ _]
          tunnel: w1185 -> [_ _ _ w1238 _ _]
          tunnel: w1182 -> [_ _ _ w1234 _ _]
          frame "Start Sequence" {
            # "Public tiff library"
            # "Get path and open file"
            n99 = Equal?(x=w1211, y=path "") -> (x = y?=w1213:bool)
            n100 = case shown="True" w1213 {
              tunnel: w1211 -> [w1215 _]
              tunnel: [w1215 w1218] -> w1210
              frame False {
              }
              frame True {
                n101 = call "File Dialog"("pattern (all files)"=".tiff", "pattern label"="Tiff Image") -> ("selected path"=w1218:path)  [unwired: 10 in, 3 out]
              }
            }
            n102 = case shown="True" "AutoIncrement" {
              tunnel: w1210 -> [w1219 w1221]
              tunnel: [w1219 w1220] -> w1206
              frame False {
              }
              frame True {
                n103 = call "4Digit File Incrementer.vi"("path"=w1221) -> ("appended path"=w1220:path)  [unwired: 10 in]
              }
            }
            n104 = local write "Path"(w1206) -> ()
            n105 = call-poly "CTIFFNewFileAndStyle.vi"("image"=w1205, "output_file"=w1206) -> ("error"=w1208:errorcluster, "CTIFF"=w1207:i64)  [unwired: 8 in]
          }
          frame "Collecting" {
            # "Add Image to write scan line"
            n106 = call-poly "CTIFFAddNewPage.vi"("error"=w1223, "image"=w1226, "CTIFF"=w1225) -> ("error"=w1222:errorcluster, "CTIFF"=w1224:i64)  [unwired: 7 in]
            n107 = property on="Ram Record" class="Bool (strict)"("DisabledEnum"=T5."Disabled and Grayed Out" ("Disabled"), "BoolText.Text"="Saving" ("Boolean Text.Text")) -> ()  [unwired: 2 in, 2 out]
          }
          frame "End" {
            (unwired) FALSE
            # "Close image file, reset capturing button"
            n108 = call "CTIFFWriteAndClose.vi"("error"=w1229, "CTIFF"=w1231) -> ("error"=w1230:errorcluster)  [unwired: 9 in]
            n109 = property on="Ram Record" class="Bool (strict)"("BoolText.Text"="RAM" ("Boolean Text.Text"), "DisabledEnum"=T5."Enabled" ("Disabled")) -> ()  [unwired: 2 in, 2 out]
          }
          frame "Read Disk" {
            n110 = call "4Digit File Incrementer tmp.vi"("Number"=w1238, "path"=path "C:/temp" ("Temp 2")) -> ("appended path"=w1236:path)  [unwired: 9 in]
            n111 = call <userlib>:"tm_opendcimgfile.vi"("Path"=w1236) -> ("Total Frames"=w1247:i32, "File Handle"=w1248:u32)  [unwired: 8 in, 1 out]
            n112 = for {
              N: w1247 -> [_]
              shift-right: [w1257] -> w1243
              shift-left: i64 0 ("CTIFF") -> [w1258]
              tunnel: [w1256] -> w1244
              tunnel: w1245 -> [w1255]
              shift-right: [w1260] -> w1239
              shift-left: w1248 -> [w1261]
              tunnel: w1235 -> [w1252]
              tunnel: w1234 -> [w1250]
              i -> [w1253]
              n113 = local write "Stack Frames"(w1253) -> ()
              n114 = Equal To 0?(x=w1253) -> (x = 0?=w1259:bool)
              n115 = call <userlib>:"tm_getdcimgframe.vi"("error in (no error)"=w1255, "Frame Index"=w1253, "File Handle in"=w1261) -> ("error out"=w1254:errorcluster, "Data"=w1249:u16[][], "File Handle out"=w1260:u32)  [unwired: 5 in, 1 out]
              n116 = call "IMAQ ArrayToImage"("Image Pixels (U16)"=w1249, "Image"=w1250) -> ("Image Out"=w1251:T1)  [unwired: 8 in, 1 out]
              n117 = case shown="True" w1259 {
                tunnel: w1249 -> [w1262 w1271]
                tunnel: w1258 -> [w1266 _]
                tunnel: [w1265 w1269] -> w1257
                tunnel: [w1264 w1267] -> w1256
                tunnel: w1254 -> [w1263 _]
                tunnel: w1252 -> [_ w1273]
                frame False {
                  n118 = call-poly "CTIFFAddNewPage.vi"("error"=w1263, "image"=w1262, "CTIFF"=w1266) -> ("error"=w1264:errorcluster, "CTIFF"=w1265:i64)  [unwired: 7 in]
                }
                frame True {
                  # "Open file dialogue is path empty"
                  # "New file doesn't\nautomatially add new page"
                  n119 = Equal?(x=w1273, y=path "") -> (x = y?=w1274:bool)
                  n120 = case shown="False" w1274 {
                    tunnel: [w1278 w1279] -> w1277
                    tunnel: w1273 -> [w1278 _]
                    frame False {
                    }
                    frame True {
                      n121 = call "File Dialog2"("pattern (all files)"=".tiff", "pattern label"="Tiff Image") -> ("selected path"=w1279:path)  [unwired: 10 in, 3 out]
                    }
                  }
                  n122 = local read "AutoIncrement"() -> (w1276:bool)
                  n123 = case shown="False" w1276 {
                    tunnel: w1277 -> [w1282 w1283]
                    tunnel: [w1282 w1284] -> w1272
                    frame False {
                    }
                    frame True {
                      n124 = call "4Digit File Incrementer.vi"("path"=w1283) -> ("appended path"=w1284:path)  [unwired: 10 in]
                    }
                  }
                  n125 = call-poly "CTIFFNewFileAndStyle.vi"("image"=w1271, "output_file"=w1272) -> ("error"=w1268:errorcluster, "CTIFF"=w1270:i64)  [unwired: 8 in]
                  n126 = local write "Path"(w1272) -> ()
                  n127 = call-poly "CTIFFAddNewPage.vi"("error"=w1268, "image"=w1271, "CTIFF"=w1270) -> ("error"=w1267:errorcluster, "CTIFF"=w1269:i64)  [unwired: 7 in]
                }
              }
              n128 = local write "Video"(w1251) -> ()
            }
            n129 = call "CTIFFWriteAndClose.vi"("error"=w1244, "CTIFF"=w1243) -> ("error"=w1241:errorcluster)  [unwired: 9 in]
            n130 = call <userlib>:"tm_closedcimgfile.vi"("error in (no error)"=w1241, "File Handle"=w1239) -> ("error out"=w1240:errorcluster)  [unwired: 9 in]
            n131 = Delete(path (use dialog)=w1236, error in=w1240) -> (error out=w1242:errorcluster)  [unwired: 3 in, 2 out]
          }
          frame "STOP" {
          }
          frame "Idle" {
          }
        }
      }
      n132 = while {
        tunnel: w18 -> [w187]
        tunnel: w21 -> [w190]
        tunnel: w32 -> [w186]
        shift-right: [w185] -> _
        shift-left: w31 -> [w188]
        shift-right: [w184] -> w27
        shift-left: w30 -> [w189]
        tunnel: w29 -> [w183]
        tunnel: [w177] -> w26
        shift-right: [w175] -> _
        shift-left: _ -> [w174]
        shift-right: [w173] -> _
        shift-left: CameraControlTypeDef."Preview" ("Enum") -> [w172]
        stop <- w176 stop-if-true
        n133 = Dequeue Element(queue=w190, timeout in ms (-1)=1) -> (element=w179:T3, timed out?=w181:bool)  [unwired: 1 in, 2 out]
        n134 = case shown="True" w181 {
          tunnel: [w191 w192] -> w180
          tunnel: w179 -> [w191 _]
          tunnel: w172 -> [_ w192]
          frame False {
          }
          frame True {
          }
        }
        n135 = case shown="\"HardDisk Record\"" w180 {
          tunnel: w189 -> [w211 w297 w361 w419 w457 w497 w534 w558 w562 w580 w591 w625 w646 w650 w671]
          tunnel: w188 -> [_ _ _ _ _ _ w538 w552 w563 _ _ _ _ w649 _]
          tunnel: w187 -> [w213 w298 _ _ _ _ _ w557 _ _ _ _ _ _ _]
          tunnel: w186 -> [w214 w281 _ _ _ _ _ w556 _ _ _ _ _ _ _]
          tunnel: [w198 w289 w374 w427 w466 w504 w538 w552 w563 w566 w589 w609 w630 w649 w654] -> w185
          tunnel: [w193 w288 w367 w425 w464 w502 w533 w551 w562 w570 w588 w621 w642 w650 w658] -> w184
          tunnel: w183 -> [w212 w296 w399 w452 w492 w512 w535 w549 w561 w583 w590 w615 w636 w651 w663]
          tunnel: [w199 w285 w373 w426 w465 w503 w532 w550 w561 w571 w587 w620 w641 w651 w659] -> w177
          tunnel: [w204 w291 w360 w418 w456 w496 w537 w548 w560 w565 w586 w607 w628 w648 w653] -> w175
          tunnel: w174 -> [w203 w291 w360 w418 w456 w496 w537 _ w560 w565 w586 w607 w628 w648 w653]
          tunnel: [w202 w290 w359 w417 w455 w495 w536 CameraControlTypeDef."Preview" ("Enum") CameraControlTypeDef."Idle" ("Enum") w564 w585 w606 w627 w647 w652] -> w173
          tunnel: w172 -> [w202 w290 w359 w417 w455 w495 w536 _ _ w564 w585 w606 w627 w647 w652]
          frame "Ram Record" {
            w197 = 1 items=["Snap", "Sequence"] ("Capture mode")
            n136 = call <userlib>:"tm_stopcapture.vi"("error in (no error)"=w212, "Handle in"=w211) -> ("error out"=w210:errorcluster, "Handle out"=w209:u32)  [unwired: 8 in]
            n137 = local read "Stacks"() -> (w196:dbl)
            n138 = call <userlib>:"tm_unpreparecapture.vi"("error in (no error)"=w210, "Handle in"=w209) -> ("error out"=w207:errorcluster, "Handle out"=w208:u32)  [unwired: 8 in]
            n139 = Flush Queue(queue=w213) -> (queue out=w206:refnum<queue>)  [unwired: 1 in, 2 out]
            n140 = for {
              N: w196 -> [_]
              tunnel: w214 -> [w235]
              tunnel: w206 -> [w227]
              tunnel: [w222] -> w205
              tunnel: [w221] -> w204
              tunnel: w203 -> [w220]
              shift-right: [w217] -> w194
              shift-left: w208 -> [w234]
              shift-right: [w215] -> w195
              shift-left: w207 -> [w233]
              w232 = 0 items=["Snap", "Sequence"] ("Capture mode")
              # "Max 2500"
              n141 = local read "Stack Frames"() -> (w223:i32)
              n142 = Bundle By Name(cluster=w235, "State"=Stack_Track."Start Sequence", "Stack Number"=0, "Image"=w220) -> (w224:T4)
              n143 = call <userlib>:"tm_preparecapture.vi"("error in (no error)"=w233, "Frames"=w223, "Capture mode"=w232, "Handle in"=w234) -> ("error out"=w231:errorcluster, "Buffer Info"=w229:T9, "Handle out"=w230:u32)  [unwired: 4 in, 1 out]
              n144 = Enqueue Element(queue=w227, element=w224) -> (queue out=w228:refnum<queue>)  [unwired: 2 in, 2 out]
              n145 = case shown="No Error" w231 {
                selector: w231 -> [w253 w270]
                tunnel: w230 -> [w252 w271]
                tunnel: w223 -> [w248 _]
                tunnel: [w237 w271] -> w218
                tunnel: w229 -> [w249 _]
                tunnel: [w236 w270] -> w216
                tunnel: w228 -> [w247 w273]
                tunnel: w235 -> [w246 _]
                tunnel: [w242 w273] -> _
                tunnel: [FALSE ("value") w275] -> _
                tunnel: [FALSE ("Boolean") _] -> w222
                tunnel: [w239 w272] -> w221
                tunnel: w220 -> [_ w272]
                frame No Error {
                  # "Frames in RAM"
                  n146 = call <userlib>:"tm_startcapture_b.vi"("error in (no error)"=w253, "Handle in"=w252) -> ("error out"=w250:errorcluster, "Handle out"=w251:u32)  [unwired: 8 in]
                  n147 = for {
                    N: w248 -> [_]
                    tunnel: w251 -> [w269]
                    tunnel: w250 -> [w268]
                    tunnel: w249 -> [w265]
                    tunnel: [w264] -> w237
                    tunnel: [w263] -> w236
                    tunnel: w247 -> [w262]
                    tunnel: Stack_Track."Collecting" ("Enum") -> [w260]
                    tunnel: w246 -> [w258]
                    tunnel: [w257] -> w244
                    tunnel: [w255] -> w239
                    tunnel: TRUE ("Boolean") -> [w254]
                    i -> [w259]
                    n148 = local write "Record Ready"(w254) -> ()
                    n149 = call <userlib>:"tm_waitnextframe.vi"("error in (no error)"=w268, "Handle in"=w269) -> ("error out"=w266:errorcluster, "Frame Index"=w256:i32, "Handle out"=w267:u32)  [unwired: 6 in, 1 out]
                    n150 = call <userlib>:"tm_getframe_a.vi"("error in (no error)"=w266, "Frame Index"=w259, "Buffer Info"=w265, "Handle in"=w267) -> ("error out"=w263:errorcluster, "Data 16"=w255:u16[][], "Handle out"=w264:u32)  [unwired: 3 in, 2 out]
                    n151 = Bundle By Name(cluster=w258, "State"=w260, "Stack Number"=w259, "Image"=w255) -> (w261:T4)
                    n152 = Enqueue Element(queue=w262, element=w261) -> (queue out=w257:refnum<queue>)  [unwired: 2 in, 2 out]
                    n153 = local write "Stack Frames"(w256) -> ()
                  }
                  n154 = Enqueue Element(queue=w244, element=T4 {"State"=enum."End", "Stack Number"=0, "Image"=[], "Stacks"=0} ("input cluster")) -> (queue out=w242:refnum<queue>)  [unwired: 2 in, 2 out]
                }
                frame Error {
                  # "Prepare camera failure, likely too many frames in stack"
                  n155 = One Button Dialog(message="Too many frames in stack", button name ("OK")="OK") -> (true=w275:bool)
                  n156 = Enqueue Element(queue=w273, element=T4 {"State"=enum."Idle", "Stack Number"=0, "Image"=[], "Stacks"=0} ("input cluster")) -> ()  [unwired: 2 in, 3 out]
                }
              }
              n157 = call <userlib>:"tm_stopcapture.vi"("error in (no error)"=w216, "Handle in"=w218) -> ("error out"=w219:errorcluster)  [unwired: 8 in, 1 out]
              n158 = call <userlib>:"tm_unpreparecapture.vi"("error in (no error)"=w219) -> ("error out"=w215:errorcluster, "Handle out"=w217:u32)  [unwired: 9 in]
            }
            n159 = local write "Record Ready"(w205) -> ()
            n160 = call <userlib>:"tm_preparecapture.vi"("error in (no error)"=w195, "Capture mode"=w197, "Handle in"=w194) -> ("error out"=w200:errorcluster, "Buffer Info"=w198:T9, "Handle out"=w201:u32)  [unwired: 5 in, 1 out]
            n161 = call <userlib>:"tm_startcapture_b.vi"("error in (no error)"=w200, "Handle in"=w201) -> ("error out"=w199:errorcluster, "Handle out"=w193:u32)  [unwired: 8 in]
          }
          frame "HardDisk Record" {
            w284 = 1 items=["Snap", "Sequence"] ("Capture mode")
            n162 = local read "Stacks"() -> (w283:dbl)
            n163 = call <userlib>:"tm_stopcapture.vi"("error in (no error)"=w296, "Handle in"=w297) -> ("error out"=w295:errorcluster, "Handle out"=w294:u32)  [unwired: 8 in]
            n164 = call <userlib>:"tm_unpreparecapture.vi"("error in (no error)"=w295, "Handle in"=w294) -> ("error out"=w292:errorcluster, "Handle out"=w293:u32)  [unwired: 8 in]
            n165 = for {
              N: w283 -> [_]
              tunnel: w298 -> [w322]
              shift-right: [w304] -> w279
              shift-left: w293 -> [w321]
              shift-right: [w305] -> w280
              shift-left: w292 -> [w320]
              tunnel: path "C:/temp" ("Temp 2") -> [w310]
              tunnel: w281 -> [w312]
              tunnel: [w299] -> w278
              i -> [w308]
              w319 = 0 items=["Snap", "Sequence"] ("Capture mode")
              # "Would add for loop here"
              # "Max 50"
              n166 = local read "Stack Frames"() -> (w316:i32)
              n167 = call "4Digit File Incrementer tmp.vi"("Number"=w308, "path"=w310) -> ("appended path"=w309:path)  [unwired: 9 in]
              n168 = call <userlib>:"tm_preparecapture.vi"("error in (no error)"=w320, "Frames"=w316, "Capture mode"=w319, "Handle in"=w321) -> ("error out"=w318:errorcluster, "Buffer Info"=w317:T9, "Handle out"=w307:u32)  [unwired: 4 in, 1 out]
              n169 = Bundle By Name(cluster=w312, "State"=Stack_Track."Read Disk", "Stack Number"=0, "Image"=u16[][] [], "Stacks"=w308) -> (w311:T4)
              n170 = case shown="No Error" w318 {
                selector: w318 -> [w330 w352]
                tunnel: w307 -> [w337 w353]
                tunnel: w317 -> [w339 _]
                tunnel: [FALSE ("value") w356] -> _
                tunnel: w316 -> [w335 _]
                tunnel: w322 -> [w333 w354]
                tunnel: w309 -> [w331 _]
                tunnel: [w329 w352] -> w301
                tunnel: [w328 w353] -> w302
                tunnel: w311 -> [w325 _]
                tunnel: TRUE ("Boolean") -> [w323 _]
                tunnel: [FALSE ("Boolean") _] -> w299
                frame No Error {
                  n171 = call <userlib>:"tm_startrecorder.vi"("error in (no error)"=w330, "frames"=w335, "File"=w331, "Handle in"=w337) -> ("error out"=w332:errorcluster, "Handle out"=w336:u32)  [unwired: 6 in]
                  n172 = call <userlib>:"tm_startcapture_b.vi"("error in (no error)"=w332, "Handle in"=w336) -> ("error out"=w340:errorcluster, "Handle out"=w341:u32)  [unwired: 8 in]
                  n173 = while {
                    tunnel: w341 -> [w349]
                    tunnel: w340 -> [w348]
                    tunnel: w339 -> [_]
                    tunnel: [w350] -> w326
                    tunnel: w335 -> [w346]
                    tunnel: [w344] -> w327
                    tunnel: w323 -> [w343]
                    i -> [w342]
                    stop <- w347 stop-if-true
                    n174 = local write "Record Ready"(w343) -> ()
                    n175 = disable-structure shown="Disabled" {
                      frame Disabled {
                        n176 = Wait (ms)(milliseconds to wait=u32 50) -> ()  [unwired: 1 out]
                      }
                      frame Enabled {
                      }
                    }
                    n177 = call <userlib>:"tm_getrecorderstatus.vi"("error in (no error)"=w348, "Handle"=w349) -> ("error out"=w350:errorcluster, "Count"=w345:i32, "Handle"=w344:u32)  [unwired: 6 in, 1 out]
                    n178 = Equal?(x=w345, y=w346) -> (x = y?=w347:bool)
                    "Stacks" <- w342
                  }
                  n179 = call <userlib>:"tm_stoprecorder.vi"("error in (no error)"=w326, "Handle in"=w327) -> ("error out"=w334:errorcluster, "Handle out"=w328:u32)  [unwired: 8 in]
                  n180 = Enqueue Element(queue=w333, element=w325, error in (no error)=w334) -> (error out=w329:errorcluster)  [unwired: 1 in, 2 out]
                }
                frame Error {
                  # "Prepare camera failure, likely too many frames in stack"
                  n181 = One Button Dialog(message="Too many frames in stack", button name ("OK")="OK") -> (true=w356:bool)
                  n182 = Enqueue Element(queue=w354, element=T4 {"State"=enum."STOP", "Stack Number"=0, "Image"=[], "Stacks"=0} ("input cluster")) -> ()  [unwired: 2 in, 3 out]
                }
              }
              n183 = call <userlib>:"tm_stopcapture.vi"("error in (no error)"=w301, "Handle in"=w302) -> ("error out"=w306:errorcluster, "Handle out"=w303:u32)  [unwired: 8 in]
              n184 = call <userlib>:"tm_unpreparecapture.vi"("error in (no error)"=w306, "Handle in"=w303) -> ("error out"=w305:errorcluster, "Handle out"=w304:u32)  [unwired: 8 in]
            }
            n185 = call <userlib>:"tm_preparecapture.vi"("error in (no error)"=w280, "Capture mode"=w284, "Handle in"=w279) -> ("error out"=w286:errorcluster, "Buffer Info"=w289:T9, "Handle out"=w287:u32)  [unwired: 5 in, 1 out]
            n186 = local write "Record Ready"(w278) -> ()
            n187 = call <userlib>:"tm_startcapture_b.vi"("error in (no error)"=w286, "Handle in"=w287) -> ("error out"=w285:errorcluster, "Handle out"=w288:u32)  [unwired: 8 in]
          }
          frame "ROI" {
            w377 = 1 items=["Snap", "Sequence"] ("Capture mode")
            n188 = call <userlib>:"tm_stopcapture.vi"("error in (no error)"=w399, "Handle in"=w361) -> ("error out"=w400:errorcluster, "Handle out"=w401:u32)  [unwired: 8 in]
            n189 = call <userlib>:"tm_unpreparecapture.vi"("error in (no error)"=w400, "Handle in"=w401) -> ("error out"=w363:errorcluster, "Handle out"=w364:u32)  [unwired: 8 in]
            n190 = local read "V Width"() -> (w369:i32)
            n191 = local read "V Offset"() -> (w371:i32)
            n192 = local read "H Width"() -> (w370:i32)
            n193 = local read "H Offset"() -> (w372:i32)
            n194 = Bundle("H Offset"=w372, "V Offset"=w371, "H Width"=w370, "V Width"=w369) -> (w368:T10)  [unwired: 1 in]
            n195 = call <userlib>:"tm_setarea.vi"("error in (no error)"=w363, "Sub Region"=w368, "Handle in"=w364) -> ("error out"=w366:errorcluster, "Handle out"=w365:u32)  [unwired: 7 in]
            n196 = call <userlib>:"tm_getarea_a.vi"("error in (no error)"=w366, "Handle in"=w365) -> ("error out"=w378:errorcluster, "V Offset"=w381:T8, "H Offset"=w382:T8, "Handle out"=w362:u32, "H Width"=w380:T8, "V Width"=w379:T8)  [unwired: 4 in]
            n197 = Unbundle By Name(w382) -> ("Value"=w386:i32, "Minimum"=w383:i32, "Maximum"=w384:i32, "Increment"=w385:i32)
            n198 = Unbundle By Name(w381) -> ("Value"=w396:i32, "Minimum"=w387:i32, "Maximum"=w388:i32, "Increment"=w389:i32)
            n199 = Unbundle By Name(w380) -> ("Value"=w397:i32, "Minimum"=w390:i32, "Maximum"=w391:i32, "Increment"=w392:i32)
            n200 = Unbundle By Name(w379) -> ("Value"=w398:i32, "Minimum"=w393:i32, "Maximum"=w394:i32, "Increment"=w395:i32)
            n201 = property on="H Offset" class="DigNum (strict)"("Value"=w386, "Minimum"=w383, "Maximum"=w384, "Increment"=w385) -> ()  [unwired: 2 in, 2 out]
            n202 = property on="V Offset" class="DigNum (strict)"("Value"=w396, "Minimum"=w387, "Maximum"=w388, "Increment"=w389) -> ()  [unwired: 2 in, 2 out]
            n203 = property on="H Width" class="DigNum (strict)"("Value"=w397, "Minimum"=w390, "Maximum"=w391, "Increment"=w392) -> ()  [unwired: 2 in, 2 out]
            n204 = property on="V Width" class="DigNum (strict)"("Value"=w398, "Minimum"=w393, "Maximum"=w394, "Increment"=w395) -> ()  [unwired: 2 in, 2 out]
            n205 = local write "SHO"(w386) -> ()
            n206 = local write "SVO"(w396) -> ()
            n207 = local write "SHW"(w397) -> ()
            n208 = local write "SVW"(w398) -> ()
            n209 = call <userlib>:"tm_preparecapture.vi"("error in (no error)"=w378, "Capture mode"=w377, "Handle in"=w362) -> ("error out"=w376:errorcluster, "Buffer Info"=w374:T9, "Handle out"=w375:u32)  [unwired: 5 in, 1 out]
            n210 = call <userlib>:"tm_startcapture_b.vi"("error in (no error)"=w376, "Handle in"=w375) -> ("error out"=w373:errorcluster, "Handle out"=w367:u32)  [unwired: 8 in]
          }
          frame "ROIWindow" {
            w430 = 1 items=["Snap", "Sequence"] ("Capture mode")
            n211 = local read "Video"() -> (w416:T1)
            n212 = call <userlib>:"tm_stopcapture.vi"("error in (no error)"=w452, "Handle in"=w419) -> ("error out"=w453:errorcluster, "Handle out"=w454:u32)  [unwired: 8 in]
            n213 = call <userlib>:"tm_unpreparecapture.vi"("error in (no error)"=w453, "Handle in"=w454) -> ("error out"=w421:errorcluster, "Handle out"=w422:u32)  [unwired: 8 in]
            n214 = call "IMAQ ConstructROI"("Image"=w416) -> ("ROI Descriptor Out"=w415:T11)  [unwired: 7 in, 3 out]
            n215 = Unbundle(w415) -> ("Contours"=w414:T12)  [unwired: 1 out]
            n216 = Index Array(array=w414, index=0) -> (element=w412:T13)
            n217 = Unbundle(w412) -> ("Coordinates"=w411:i32[])  [unwired: 2 out]
            n218 = Index Array(array=w411, index #1=0 ("index"), index #2=1 ("index"), index #3=2 ("index"), index #4=3 ("index")) -> (element #1=w406:i32, element #2=w405:i32, element #3=w404:i32, element #4=w403:i32)
            n219 = Bundle(w406, w405, w404, w403) -> (w402:cluster{i32, i32, i32, i32})  [unwired: 1 in]
            n220 = call <userlib>:"tm_setarea.vi"("error in (no error)"=w421, "Sub Region"=w402, "Handle in"=w422) -> ("error out"=w424:errorcluster, "Handle out"=w423:u32)  [unwired: 7 in]
            n221 = call <userlib>:"tm_getarea_a.vi"("error in (no error)"=w424, "Handle in"=w423) -> ("error out"=w431:errorcluster, "V Offset"=w434:T8, "H Offset"=w435:T8, "Handle out"=w420:u32, "H Width"=w433:T8, "V Width"=w432:T8)  [unwired: 4 in]
            n222 = Unbundle By Name(w435) -> ("Value"=w439:i32, "Minimum"=w436:i32, "Maximum"=w437:i32, "Increment"=w438:i32)
            n223 = Unbundle By Name(w434) -> ("Value"=w449:i32, "Minimum"=w440:i32, "Maximum"=w441:i32, "Increment"=w442:i32)
            n224 = Unbundle By Name(w433) -> ("Value"=w450:i32, "Minimum"=w443:i32, "Maximum"=w444:i32, "Increment"=w445:i32)
            n225 = Unbundle By Name(w432) -> ("Value"=w451:i32, "Minimum"=w446:i32, "Maximum"=w447:i32, "Increment"=w448:i32)
            n226 = property on="H Offset" class="DigNum (strict)"("Value"=w439, "Minimum"=w436, "Maximum"=w437, "Increment"=w438) -> ()  [unwired: 2 in, 2 out]
            n227 = property on="V Offset" class="DigNum (strict)"("Value"=w449, "Minimum"=w440, "Maximum"=w441, "Increment"=w442) -> ()  [unwired: 2 in, 2 out]
            n228 = property on="H Width" class="DigNum (strict)"("Value"=w450, "Minimum"=w443, "Maximum"=w444, "Increment"=w445) -> ()  [unwired: 2 in, 2 out]
            n229 = property on="V Width" class="DigNum (strict)"("Value"=w451, "Minimum"=w446, "Maximum"=w447, "Increment"=w448) -> ()  [unwired: 2 in, 2 out]
            n230 = local write "SHO"(w439) -> ()
            n231 = local write "SVO"(w449) -> ()
            n232 = local write "SHW"(w450) -> ()
            n233 = local write "SVW"(w451) -> ()
            n234 = call <userlib>:"tm_preparecapture.vi"("error in (no error)"=w431, "Capture mode"=w430, "Handle in"=w420) -> ("error out"=w429:errorcluster, "Buffer Info"=w427:T9, "Handle out"=w428:u32)  [unwired: 5 in, 1 out]
            n235 = call <userlib>:"tm_startcapture_b.vi"("error in (no error)"=w429, "Handle in"=w428) -> ("error out"=w426:errorcluster, "Handle out"=w425:u32)  [unwired: 8 in]
          }
          frame "Binning" {
            w469 = 1 items=["Snap", "Sequence"] ("Capture mode")
            w459 = u32 4215968 items=["BINNING"=4215968, "BITS PER CHANNEL"=2, "ACTIVE VIEW INDEX"=3, "CCD MODE"=4, "SENSOR MODE"=5, "READOUT MODE"=6, "EXPOSURE TIME"=7, "CONTRAST GAIN"=8, "CONTRAST OFFSET"=9, "LIGHT MODE"=10, "SENSITIVITY"=11, "WHITE BALANCE"=12, "PHOTON IMAGING MODE"=13, "HIGH DYNAMIC RANGE MODE"=14, "TRIGGER SOURCE"=15, "TRIGGER ACTIVE"=16, "TRIGGER MODE"=17, "TRIGGER POLARITY"=18, "TRIGGER GLOBAL EXPOSURE"=19, "FIRST TRIGGER BEHAVIOR"=20, "TRIGGER TIMES"=21, "OUTPUT TRIGGER POLARITY"=22, "OUTPUT TRIGGER DELAY"=23, "OUTPUT TRIGGER PERIOD"=24, "TEMPERATURE"=25, "TEMPERATURE TARGET"=26, "SENSOR COOLER FAN"=27, "MECHANICAL SHUTTER"=28, "BACK FOCUS POSITION"=29, "FRAMEBUNDLE MODE"=30, "FRAMEBUNDLE NUMBER"=31, "LINEBUNDLE HEIGHT"=32, "TRIGGER CONNECTOR"=33, "IMAGE PIXEL TYPE"=34, "OUTPUT TRIGGER KIND"=35, "READOUT DIRECTION"=36, "CHANNEL SYNC"=37] ("Parameter")
            n236 = local read "Binning"() -> (w491:u16)
            n237 = call <userlib>:"tm_stopcapture.vi"("error in (no error)"=w492, "Handle in"=w457) -> ("error out"=w493:errorcluster, "Handle out"=w494:u32)  [unwired: 8 in]
            n238 = call <userlib>:"tm_unpreparecapture.vi"("error in (no error)"=w493, "Handle in"=w494) -> ("error out"=w462:errorcluster, "Handle out"=w463:u32)  [unwired: 8 in]
            n239 = call <userlib>:"tm_setparameter_a.vi"("error in (no error)"=w462, "Value in"=w491, "Parameter"=w459, "Handle in"=w463) -> ("error out"=w460:errorcluster, "Handle out"=w458:u32)  [unwired: 6 in]
            n240 = call <userlib>:"tm_getarea_a.vi"("error in (no error)"=w460, "Handle in"=w458) -> ("error out"=w470:errorcluster, "V Offset"=w473:T8, "H Offset"=w474:T8, "Handle out"=w461:u32, "H Width"=w472:T8, "V Width"=w471:T8)  [unwired: 4 in]
            n241 = Unbundle By Name(w474) -> ("Value"=w478:i32, "Minimum"=w475:i32, "Maximum"=w476:i32, "Increment"=w477:i32)
            n242 = Unbundle By Name(w473) -> ("Value"=w488:i32, "Minimum"=w479:i32, "Maximum"=w480:i32, "Increment"=w481:i32)
            n243 = Unbundle By Name(w472) -> ("Value"=w489:i32, "Minimum"=w482:i32, "Maximum"=w483:i32, "Increment"=w484:i32)
            n244 = Unbundle By Name(w471) -> ("Value"=w490:i32, "Minimum"=w485:i32, "Maximum"=w486:i32, "Increment"=w487:i32)
            n245 = property on="H Offset" class="DigNum (strict)"("Value"=w478, "Minimum"=w475, "Maximum"=w476, "Increment"=w477) -> ()  [unwired: 2 in, 2 out]
            n246 = property on="V Offset" class="DigNum (strict)"("Value"=w488, "Minimum"=w479, "Maximum"=w480, "Increment"=w481) -> ()  [unwired: 2 in, 2 out]
            n247 = property on="H Width" class="DigNum (strict)"("Value"=w489, "Minimum"=w482, "Maximum"=w483, "Increment"=w484) -> ()  [unwired: 2 in, 2 out]
            n248 = property on="V Width" class="DigNum (strict)"("Value"=w490, "Minimum"=w485, "Maximum"=w486, "Increment"=w487) -> ()  [unwired: 2 in, 2 out]
            n249 = local write "SHO"(w478) -> ()
            n250 = local write "SVO"(w488) -> ()
            n251 = local write "SHW"(w489) -> ()
            n252 = local write "SVW"(w490) -> ()
            n253 = call <userlib>:"tm_preparecapture.vi"("error in (no error)"=w470, "Capture mode"=w469, "Handle in"=w461) -> ("error out"=w468:errorcluster, "Buffer Info"=w466:T9, "Handle out"=w467:u32)  [unwired: 5 in, 1 out]
            n254 = call <userlib>:"tm_startcapture_b.vi"("error in (no error)"=w468, "Handle in"=w467) -> ("error out"=w465:errorcluster, "Handle out"=w464:u32)  [unwired: 8 in]
          }
          frame "Readout Mode" {
            w507 = 1 items=["Snap", "Sequence"] ("Capture mode")
            # "Set mode to Light Shheet\nUse 12"
            # "Currently only uses auto calculate. \nAleks would probably use manual. Add option."
            n255 = call <userlib>:"tm_stopcapture.vi"("error in (no error)"=w512, "Handle in"=w497) -> ("error out"=w513:errorcluster, "Handle out"=w514:u32)  [unwired: 8 in]
            n256 = call <userlib>:"tm_unpreparecapture.vi"("error in (no error)"=w513, "Handle in"=w514) -> ("error out"=w498:errorcluster, "Handle out"=w499:u32)  [unwired: 8 in]
            n257 = local read "Camera Readout Mode"() -> (w510:u16)
            n258 = call <userlib>:"tm_setpropertyvalue.vi"("error in (no error)"=w498, "Value in"=w510, "Property ID"=u32 4194832, "Handle in"=w499) -> ("error out"=w508:errorcluster, "Handle out"=w509:u32)  [unwired: 6 in]
            n259 = case shown="12" w510 {
              tunnel: [w518 w523] -> w501
              tunnel: w509 -> [w517 w524]
              tunnel: w508 -> [w516 w523]
              tunnel: [w515 w522] -> w500
              frame 1, Default {
                n260 = local read "Exposure"() -> (w519:dbl)
                n261 = call <userlib>:"tm_setpropertyvalue.vi"("error in (no error)"=w516, "Value in"=w519, "Property ID"=u32 2031888, "Handle in"=w517) -> ("error out"=w518:errorcluster, "Handle out"=w515:u32)  [unwired: 6 in]
              }
              frame 12 {
                # "Aleks uses 10e-6"
                n262 = local read "Slit Width / Lines"() -> (w521:sgl)
                n263 = local read "Exposure"() -> (w531:dbl)
                n264 = local read "SVW"() -> (w530:i32)
                n265 = formula code="slitExpos=frameInter*LW/(LinesToReadout\n+10+LW);\nlineInter = slitExpos / LW;"("frameInter"=w531, "LW"=w521, "LinesToReadout"=w530) -> ("slitExpos"=w525:dbl, "lineInter"=w528:dbl)
                "Internal Line Interval" <- w528
                n266 = call <userlib>:"tm_setpropertyvalue.vi"("Value in"=w528, "Property ID"=u32 4208720, "Handle in"=w524) -> ("Handle out"=w527:u32)  [unwired: 7 in, 1 out]
                n267 = call <userlib>:"tm_setpropertyvalue.vi"("Value in"=w525, "Property ID"=u32 2031888, "Handle in"=w527) -> ("Handle out"=w522:u32)  [unwired: 7 in, 1 out]
              }
            }
            n268 = call <userlib>:"tm_preparecapture.vi"("error in (no error)"=w501, "Capture mode"=w507, "Handle in"=w500) -> ("error out"=w506:errorcluster, "Buffer Info"=w504:T9, "Handle out"=w505:u32)  [unwired: 5 in, 1 out]
            n269 = call <userlib>:"tm_startcapture_b.vi"("error in (no error)"=w506, "Handle in"=w505) -> ("error out"=w503:errorcluster, "Handle out"=w502:u32)  [unwired: 8 in]
          }
          frame "Update" {
            w539 = u32 2049184 items=["SENSOR MODE"=4212128, "CCD MODE"=4212384, "READOUT MODE"=4211872, "ACTIVE VIEW INDEX"=4343136, "BITS PER CHANNEL"=4342976, "IMAGE PIXEL TYPE"=4343296, "BINNING"=4215968, "EXPOSURE TIME"=2049184, "CONTRAST GAIN"=3163312, "CONTRAST OFFSET"=3163328, "LIGHT MODE"=2114720, "SENSITIVITY"=2114992, "PHOTON IMAGING MODE"=2115200, "HIGH DYNAMIC RANGE MODE"=3163360, "WHITE BALANCE"=3163568, "TEMPERATURE"=2115232, "TEMPERATURE TARGET"=2115264, "SENSOR COOLER FAN"=2115296, "LINEBUNDLE HEIGHT"=4212192, "MECHANICAL SHUTTER"=2115488, "BACK FOCUS POSITION"=8422304, "TRIGGER CONNECTOR"=1066432, "TRIGGER SOURCE"=1066144, "OUTPUT TRIGGER SOURCE"=1852576, "TRIGGER GLOBAL EXPOSURE"=2049680, "FIRST TRIGGER BEHAVIOR"=2049696, "CHANNEL SYNC"=1852352, "READOUT DIRECTION"=4211904, "PRE HSYNC COUNT"=1852704] ("Parameter")
            # "Error on get"
            n270 = local read "Exposure"() -> (w541:dbl)
            n271 = call <userlib>:"tm_setparameter_a.vi"("error in (no error)"=w535, "Value in"=w541, "Parameter"=w539, "Handle in"=w534) -> ("error out"=w543:errorcluster, "Handle out"=w540:u32)  [unwired: 6 in]
            n272 = call <userlib>:"tm_getparameter_a.vi"("error in (no error)"=w543, "Parameter"=w539, "Handle in"=w540) -> ("error out"=w532:errorcluster, "Value out"=w542:dbl, "Handle out"=w533:u32)  [unwired: 6 in]
            n273 = local write "EXP"(w542) -> ()
          }
          frame "Preview", Default {
            # "Slows it all down somewhat"
            # "Currently the external trigger setting means that frames are dropped because the system lingers at this point. \nIdeally I should set it so when the system is external and recording it won't run this section.\n\nThis is what HC Image does, it offers no live video when you switch from live to record mode.\n\nRealistically when tirgger set external and this times out once then ignore this step.\nBut it'd have to be reset after a recording.\n\nNeed to think more betterer about how to handle this else frames will just be dropped. Probably best to just have a seperate scan mode\nOr at least just a boolean to turn off this live capture section. Working now maybe"
            n274 = call <userlib>:"tm_waitnextframe.vi"("error in (no error)"=w549, "Timeout"=3000, "Handle in"=w558) -> ("error out"=w545:errorcluster, "Handle out"=w546:u32)  [unwired: 5 in, 2 out]
            n275 = call <userlib>:"tm_getframe_a.vi"("error in (no error)"=w545, "Buffer Info"=w552, "Handle in"=w546) -> ("error out"=w550:errorcluster, "Data 16"=w548:u16[][], "Handle out"=w551:u32)  [unwired: 4 in, 2 out]
            n276 = Bundle By Name(cluster=w556, "State"=Stack_Track."Idle", "Stack Number"=0, "Image"=w548) -> (w553:T4)
            n277 = Enqueue Element(queue=w557, element=w553) -> ()  [unwired: 2 in, 3 out]
          }
          frame "Idle" {
          }
          frame "Scan Mode" {
            w567 = 1 items=["Snap", "Sequence"] ("Capture mode")
            w576 = u32 4211872 items=["SENSOR MODE"=4212128, "CCD MODE"=4212384, "READOUT MODE"=4211872, "ACTIVE VIEW INDEX"=4343136, "BITS PER CHANNEL"=4342976, "IMAGE PIXEL TYPE"=4343296, "BINNING"=4215968, "EXPOSURE TIME"=2049184, "CONTRAST GAIN"=3163312, "CONTRAST OFFSET"=3163328, "LIGHT MODE"=2114720, "SENSITIVITY"=2114992, "PHOTON IMAGING MODE"=2115200, "HIGH DYNAMIC RANGE MODE"=3163360, "WHITE BALANCE"=3163568, "TEMPERATURE"=2115232, "TEMPERATURE TARGET"=2115264, "SENSOR COOLER FAN"=2115296, "LINEBUNDLE HEIGHT"=4212192, "MECHANICAL SHUTTER"=2115488, "BACK FOCUS POSITION"=8422304, "TRIGGER CONNECTOR"=1066432, "TRIGGER SOURCE"=1066144, "OUTPUT TRIGGER SOURCE"=1852576, "TRIGGER GLOBAL EXPOSURE"=2049680, "FIRST TRIGGER BEHAVIOR"=2049696, "CHANNEL SYNC"=1852352, "READOUT DIRECTION"=4211904, "PRE HSYNC COUNT"=1852704] ("Parameter")
            n278 = call <userlib>:"tm_stopcapture.vi"("error in (no error)"=w583, "Handle in"=w580) -> ("error out"=w582:errorcluster, "Handle out"=w581:u32)  [unwired: 8 in]
            n279 = call <userlib>:"tm_unpreparecapture.vi"("error in (no error)"=w582, "Handle in"=w581) -> ("error out"=w578:errorcluster, "Handle out"=w579:u32)  [unwired: 8 in]
            n280 = local read "Scan Mode"() -> (w577:dbl)
            n281 = call <userlib>:"tm_setparameter_a.vi"("error in (no error)"=w578, "Value in"=w577, "Parameter"=w576, "Handle in"=w579) -> ("error out"=w572:errorcluster)  [unwired: 6 in, 1 out]
            n282 = call <userlib>:"tm_getparameter_a.vi"("error in (no error)"=w572, "Parameter"=w576) -> ("error out"=w573:errorcluster, "Value out"=w575:dbl, "Handle out"=w568:u32)  [unwired: 7 in]
            n283 = local write "SMD"(w575) -> ()
            n284 = call <userlib>:"tm_preparecapture.vi"("error in (no error)"=w573, "Capture mode"=w567, "Handle in"=w568) -> ("error out"=w574:errorcluster, "Buffer Info"=w566:T9, "Handle out"=w569:u32)  [unwired: 5 in, 1 out]
            n285 = call <userlib>:"tm_startcapture_b.vi"("error in (no error)"=w574, "Handle in"=w569) -> ("error out"=w571:errorcluster, "Handle out"=w570:u32)  [unwired: 8 in]
          }
          frame "Trigger Mode" {
            w584 = 1 items=["Snap", "Sequence"] ("Capture mode")
            w592 = u32 1049104 ("Property ID")
            n286 = local read "Trigger Mode"() -> (w597:sgl)
            n287 = call <userlib>:"tm_stopcapture.vi"("error in (no error)"=w590, "Handle in"=w591) -> ("error out"=w596:errorcluster, "Handle out"=w604:u32)  [unwired: 8 in]
            n288 = call <userlib>:"tm_unpreparecapture.vi"("error in (no error)"=w596, "Handle in"=w604) -> ("error out"=w594:errorcluster, "Handle out"=w600:u32)  [unwired: 8 in]
            n289 = call <userlib>:"tm_setpropertyvalue.vi"("error in (no error)"=w594, "Value in"=w597, "Property ID"=w592, "Handle in"=w600) -> ("error out"=w593:errorcluster, "Handle out"=w599:u32)  [unwired: 6 in]
            n290 = call <userlib>:"tm_getpropertyvalue.vi"("error in (no error)"=w593, "Property ID"=w592, "Handle in"=w599) -> ("error out"=w601:errorcluster, "Value in"=w598:sgl, "Handle out"=w602:u32)  [unwired: 6 in]
            n291 = local write "Trigger Mode"(w598) -> ()
            n292 = call <userlib>:"tm_preparecapture.vi"("error in (no error)"=w601, "Capture mode"=w584, "Handle in"=w602) -> ("error out"=w595:errorcluster, "Buffer Info"=w589:T9, "Handle out"=w603:u32)  [unwired: 5 in, 1 out]
            n293 = call <userlib>:"tm_startcapture_b.vi"("error in (no error)"=w595, "Handle in"=w603) -> ("error out"=w587:errorcluster, "Handle out"=w588:u32)  [unwired: 8 in]
          }
          frame "Readout Direction" {
            w605 = u32 4211904 items=["SENSOR MODE"=4212128, "CCD MODE"=4212384, "READOUT MODE"=4211872, "ACTIVE VIEW INDEX"=4343136, "BITS PER CHANNEL"=4342976, "IMAGE PIXEL TYPE"=4343296, "BINNING"=4215968, "EXPOSURE TIME"=2049184, "CONTRAST GAIN"=3163312, "CONTRAST OFFSET"=3163328, "LIGHT MODE"=2114720, "SENSITIVITY"=2114992, "PHOTON IMAGING MODE"=2115200, "HIGH DYNAMIC RANGE MODE"=3163360, "WHITE BALANCE"=3163568, "TEMPERATURE"=2115232, "TEMPERATURE TARGET"=2115264, "SENSOR COOLER FAN"=2115296, "LINEBUNDLE HEIGHT"=4212192, "MECHANICAL SHUTTER"=2115488, "BACK FOCUS POSITION"=8422304, "TRIGGER CONNECTOR"=1066432, "TRIGGER SOURCE"=1066144, "OUTPUT TRIGGER SOURCE"=1852576, "TRIGGER GLOBAL EXPOSURE"=2049680, "FIRST TRIGGER BEHAVIOR"=2049696, "CHANNEL SYNC"=1852352, "READOUT DIRECTION"=4211904, "PRE HSYNC COUNT"=1852704, "INTERNAL LINE SPEED"=4226000, "INTERNAL LINE INTERVAL"=4226016] ("Parameter")
            w616 = 1 items=["Snap", "Sequence"] ("Capture mode")
            n294 = call <userlib>:"tm_stopcapture.vi"("error in (no error)"=w615, "Handle in"=w625) -> ("error out"=w617:errorcluster, "Handle out"=w624:u32)  [unwired: 8 in]
            n295 = call <userlib>:"tm_unpreparecapture.vi"("error in (no error)"=w617, "Handle in"=w624) -> ("error out"=w618:errorcluster, "Handle out"=w623:u32)  [unwired: 8 in]
            n296 = local read "Readout Direction"() -> (w608:sgl)
            n297 = call <userlib>:"tm_setparameter_a.vi"("error in (no error)"=w618, "Value in"=w608, "Parameter"=w605, "Handle in"=w623) -> ("error out"=w612:errorcluster, "Handle out"=w614:u32)  [unwired: 6 in]
            n298 = call <userlib>:"tm_getparameter_a.vi"("error in (no error)"=w612, "Parameter"=w605, "Handle in"=w614) -> ("error out"=w611:errorcluster, "Value out"=w610:dbl, "Handle out"=w613:u32)  [unwired: 6 in]
            n299 = local write "Readout Direction"(w610) -> ()
            n300 = call <userlib>:"tm_preparecapture.vi"("error in (no error)"=w611, "Capture mode"=w616, "Handle in"=w613) -> ("error out"=w619:errorcluster, "Buffer Info"=w609:T9, "Handle out"=w622:u32)  [unwired: 5 in, 1 out]
            n301 = call <userlib>:"tm_startcapture_b.vi"("error in (no error)"=w619, "Handle in"=w622) -> ("error out"=w620:errorcluster, "Handle out"=w621:u32)  [unwired: 8 in]
          }
          frame "IntervalLineInt" {
            w626 = 4226016
            w637 = 1 items=["Snap", "Sequence"] ("Capture mode")
            n302 = call <userlib>:"tm_stopcapture.vi"("error in (no error)"=w636, "Handle in"=w646) -> ("error out"=w638:errorcluster, "Handle out"=w645:u32)  [unwired: 8 in]
            n303 = call <userlib>:"tm_unpreparecapture.vi"("error in (no error)"=w638, "Handle in"=w645) -> ("error out"=w639:errorcluster, "Handle out"=w644:u32)  [unwired: 8 in]
            n304 = local read "Internal Line Interval"() -> (w629:dbl)
            n305 = call <userlib>:"tm_setparameter_a.vi"("error in (no error)"=w639, "Value in"=w629, "Parameter"=w626, "Handle in"=w644) -> ("error out"=w633:errorcluster, "Handle out"=w635:u32)  [unwired: 6 in]
            n306 = call <userlib>:"tm_getparameter_a.vi"("error in (no error)"=w633, "Parameter"=w626, "Handle in"=w635) -> ("error out"=w632:errorcluster, "Value out"=w631:dbl, "Handle out"=w634:u32)  [unwired: 6 in]
            n307 = local write "Internal Line Interval"(w631) -> ()
            n308 = call <userlib>:"tm_preparecapture.vi"("error in (no error)"=w632, "Capture mode"=w637, "Handle in"=w634) -> ("error out"=w640:errorcluster, "Buffer Info"=w630:T9, "Handle out"=w643:u32)  [unwired: 5 in, 1 out]
            n309 = call <userlib>:"tm_startcapture_b.vi"("error in (no error)"=w640, "Handle in"=w643) -> ("error out"=w641:errorcluster, "Handle out"=w642:u32)  [unwired: 8 in]
          }
          frame "Disengage Update" {
          }
          frame "Trigger Source" {
            w655 = 1 items=["Snap", "Sequence"] ("Capture mode")
            w666 = u32 1066144 items=["SENSOR MODE"=4212128, "CCD MODE"=4212384, "READOUT MODE"=4211872, "ACTIVE VIEW INDEX"=4343136, "BITS PER CHANNEL"=4342976, "IMAGE PIXEL TYPE"=4343296, "BINNING"=4215968, "EXPOSURE TIME"=2049184, "CONTRAST GAIN"=3163312, "CONTRAST OFFSET"=3163328, "LIGHT MODE"=2114720, "SENSITIVITY"=2114992, "PHOTON IMAGING MODE"=2115200, "HIGH DYNAMIC RANGE MODE"=3163360, "WHITE BALANCE"=3163568, "TEMPERATURE"=2115232, "TEMPERATURE TARGET"=2115264, "SENSOR COOLER FAN"=2115296, "LINEBUNDLE HEIGHT"=4212192, "MECHANICAL SHUTTER"=2115488, "BACK FOCUS POSITION"=8422304, "TRIGGER CONNECTOR"=1066432, "TRIGGER SOURCE"=1066144, "OUTPUT TRIGGER SOURCE"=1852576, "TRIGGER GLOBAL EXPOSURE"=2049680, "FIRST TRIGGER BEHAVIOR"=2049696, "CHANNEL SYNC"=1852352, "READOUT DIRECTION"=4211904, "PRE HSYNC COUNT"=1852704, "INTERNAL LINE SPEED"=4226000, "INTERNAL LINE INTERVAL"=4226016] ("Parameter")
            n310 = call <userlib>:"tm_stopcapture.vi"("error in (no error)"=w663, "Handle in"=w671) -> ("error out"=w672:errorcluster, "Handle out"=w670:u32)  [unwired: 8 in]
            n311 = call <userlib>:"tm_unpreparecapture.vi"("error in (no error)"=w672, "Handle in"=w670) -> ("error out"=w664:errorcluster, "Handle out"=w669:u32)  [unwired: 8 in]
            n312 = local read "Trigger Source"() -> (w668:sgl)
            n313 = call <userlib>:"tm_setparameter_a.vi"("error in (no error)"=w664, "Value in"=w668, "Parameter"=w666, "Handle in"=w669) -> ("error out"=w662:errorcluster, "Handle out"=w667:u32)  [unwired: 6 in]
            n314 = call <userlib>:"tm_getparameter_a.vi"("error in (no error)"=w662, "Parameter"=w666, "Handle in"=w667) -> ("error out"=w661:errorcluster, "Value out"=w665:dbl, "Handle out"=w656:u32)  [unwired: 6 in]
            n315 = local write "Trigger Source"(w665) -> ()
            n316 = call <userlib>:"tm_preparecapture.vi"("error in (no error)"=w661, "Capture mode"=w655, "Handle in"=w656) -> ("error out"=w660:errorcluster, "Buffer Info"=w654:T9, "Handle out"=w657:u32)  [unwired: 5 in, 1 out]
            n317 = call <userlib>:"tm_startcapture_b.vi"("error in (no error)"=w660, "Handle in"=w657) -> ("error out"=w659:errorcluster, "Handle out"=w658:u32)  [unwired: 8 in]
          }
        }
        n318 = local read "stop"() -> (w178:bool)
        n319 = Compound Arithmetic op=OR(w178, w177) -> (w176:bool)
      }
      n320 = disable-structure shown="Disabled" {
        disable-tunnel: 0.0 -> [w682 _]
        disable-tunnel: w97 -> [w681 _]
        disable-tunnel: 0 -> [w680 _]
        disable-tunnel: [w679 _] -> _
        disable-tunnel: [w678 _] -> _
        disable-tunnel: w32 -> [w677 _]
        disable-tunnel: w31 -> [w676 _]
        disable-tunnel: w30 -> [w675 _]
        disable-tunnel: w29 -> [w674 _]
        disable-tunnel: w18 -> [w673 _]
        frame Disabled {
          n321 = while {
            tunnel: w674 -> [w696]
            tunnel: [w694] -> w678
            tunnel: [w693] -> w679
            shift-right: [w703] -> _
            shift-left: w681 -> [w701]
            shift-right: [w704] -> _
            shift-left: w682 -> [w702]
            shift-right: [w695] -> _
            shift-left: w681 -> [w699]
            tunnel: w675 -> [w697]
            tunnel: w681 -> [w700]
            shift-right: [w692] -> _
            shift-left: w676 -> [w698]
            shift-right: [w690] -> _
            shift-left: w680 -> [w691]
            tunnel: w673 -> [w689]
            shift-right: [w687] -> _
            shift-left: _ -> [w686]
            tunnel: w677 -> [w685]
            stop <- w705 stop-if-true
            n322 = event shown="[8] \"HardDisk Record\": Value Change" {
              selector: _ -> [_ _ _ _ _ _ _ _ _ _ _ _]
              dyn-events: _ -> [_ _ _ _ _ _ _ _ _ _ _ _]
              timeout: 0 -> [_ _ _ _ _ _ _ _ _ _ _ _]
              tunnel: [w716 w785 w799 w812 w831 w851 w873 w901 w998 w1092 w1128 w1173] -> w704
              tunnel: [w715 w786 w800 w813 w832 w852 w874 w902 w999 w1093 w1129 w1174] -> w703
              tunnel: w702 -> [w727 w785 w799 w812 w831 w851 w873 w901 w998 w1092 w1128 w1173]
              tunnel: w701 -> [w718 w786 w800 w813 w832 w852 w874 w902 w999 w1093 w1129 w1174]
              tunnel: w700 -> [w723 _ _ _ _ _ _ _ _ _ _ _]
              tunnel: w699 -> [w728 w787 w801 w814 w833 w853 w875 w897 w994 w1094 w1136 w1181]
              tunnel: w698 -> [w722 w784 w798 w811 _ w850 _ w898 w995 _ _ _]
              tunnel: w697 -> [w730 w780 w793 w807 w826 w844 w866 w905 w1002 w1089 w1105 w1143]
              tunnel: w696 -> [w729 w782 w789 w808 w825 w847 w865 w906 w1003 w1088 w1104 w1142]
              tunnel: [w726 w787 w801 w814 w833 w853 w875 w897 w994 w1094 w1136 w1181] -> w695
              tunnel: [w725 w777 w796 w804 w817 w837 w856 w903 w1000 w1083 w1131 w1176] -> w694
              tunnel: [w724 w776 w795 w803 w816 w836 w854 w904 w1001 w1084 w1132 w1177] -> w693
              tunnel: [w721 w784 w798 w811 w820 w850 w861 w899 w996 w1082 w1130 w1175] -> w692
              tunnel: w691 -> [w713 w783 w797 w810 w830 w849 w872 w900 w997 w1081 w1101 w1137]
              tunnel: [w712 w783 w797 w810 w830 w849 w872 w900 w997 w1081 w1101 w1137] -> w690
              tunnel: w689 -> [w707 _ _ _ _ _ _ w896 w993 _ _ _]
              tunnel: [_ _ _ _ _ _ _ w895 w992 _ _ _] -> w688
              tunnel: w685 -> [w710 _ _ _ _ _ _ w893 _ _ _ _]
              tunnel: [w709 _ _ _ _ _ _ _ _ _ _ _] -> w687
              tunnel: w686 -> [w708 _ _ _ _ _ _ w894 _ _ _ _]
              event Timeout {
                n323 = event-data() -> ()  [unwired: 1 in, 2 out]
                n324 = call <userlib>:"tm_waitnextframe.vi"("error in (no error)"=w729, "Handle in"=w730) -> ("error out"=w733:errorcluster, "Frame Count"=w714:i32, "Frame Index"=w732:i32, "Handle out"=w734:u32)  [unwired: 6 in]
                "Total Frames" <- w714
                n325 = Tick Count (ms)() -> (millisecond timer value=w720:u32)
                n326 = Increment(x=w727) -> (x+1=w717:dbl)
                n327 = Subtract(x=w720, y=w723) -> (x-y=→"Elapsed Time":u32)
                n328 = Add(x=w718, y=u32 1000) -> (x+y=w738:u32)
                n329 = Less Or Equal?(x=w738, y=w720) -> (x <= y?=w719:bool)
                n330 = Add(x=w728, y=u32 50) -> (x+y=w736:u32)
                n331 = Less Or Equal?(x=w736, y=w720) -> (x <= y?=w711:bool)
                n332 = case shown="True" w719 {
                  tunnel: w718 -> [w741 w750]
                  tunnel: [w741 w747] -> w715
                  tunnel: w717 -> [w740 w753]
                  tunnel: w720 -> [_ w747]
                  tunnel: [w740 0.0] -> w716
                  tunnel: w714 -> [_ w742]
                  tunnel: w713 -> [w739 w745]
                  tunnel: [w739 w742] -> w712
                  frame False {
                  }
                  frame True {
                    n333 = Subtract(x=w747, y=w750) -> (x-y=w749:u32)
                    n334 = Subtract(x=w742, y=w745) -> (x-y=w743:i32)
                    n335 = To Double Precision Float(number=w749) -> (double precision float=w755:dbl)
                    n336 = Divide(x=w755, y=1000.0) -> (x/y=w746:dbl)
                    n337 = To Double Precision Float(number=w743) -> (double precision float=w744:dbl)
                    n338 = Divide(x=w744, y=w746) -> (x/y=→"Camera FPS":dbl)
                    n339 = Divide(x=w753, y=w746) -> (x/y=→"Software FPS":dbl)
                  }
                }
                n340 = case shown="True" w711 {
                  tunnel: w728 -> [w760 _]
                  tunnel: w720 -> [_ w773]
                  tunnel: [w760 w773] -> w726
                  tunnel: w734 -> [w759 w772]
                  tunnel: w722 -> [w757 w767]
                  tunnel: w733 -> [w758 w771]
                  tunnel: [w759 w770] -> w725
                  tunnel: [w758 w769] -> w724
                  tunnel: w732 -> [_ w768]
                  tunnel: [w757 w767] -> w721
                  tunnel: w707 -> [_ w766]
                  tunnel: w710 -> [_ w762]
                  tunnel: [w756 w761] -> w709
                  tunnel: w708 -> [w756 _]
                  frame False {
                  }
                  frame True {
                    n341 = call <userlib>:"tm_getframe_a.vi"("error in (no error)"=w771, "Frame Index"=w768, "Buffer Info"=w767, "Handle in"=w772) -> ("error out"=w769:errorcluster, "Data 16"=w761:u16[][], "Handle out"=w770:u32)  [unwired: 3 in, 2 out]
                    n342 = Bundle By Name(cluster=w762, "State"=Stack_Track."Idle", "Stack Number"=0, "Image"=w761) -> (w763:T4)
                    n343 = Enqueue Element(queue=w766, element=w763) -> ()  [unwired: 2 in, 3 out]
                  }
                }
              }
              event "Exposure": Value Change {
                w775 = u32 2049184 items=["SENSOR MODE"=4212128, "CCD MODE"=4212384, "READOUT MODE"=4211872, "ACTIVE VIEW INDEX"=4343136, "BITS PER CHANNEL"=4342976, "IMAGE PIXEL TYPE"=4343296, "BINNING"=4215968, "EXPOSURE TIME"=2049184, "CONTRAST GAIN"=3163312, "CONTRAST OFFSET"=3163328, "LIGHT MODE"=2114720, "SENSITIVITY"=2114992, "PHOTON IMAGING MODE"=2115200, "HIGH DYNAMIC RANGE MODE"=3163360, "WHITE BALANCE"=3163568, "TEMPERATURE"=2115232, "TEMPERATURE TARGET"=2115264, "SENSOR COOLER FAN"=2115296, "LINEBUNDLE HEIGHT"=4212192, "MECHANICAL SHUTTER"=2115488, "BACK FOCUS POSITION"=8422304, "TRIGGER CONNECTOR"=1066432, "TRIGGER SOURCE"=1066144, "OUTPUT TRIGGER SOURCE"=1852576, "TRIGGER GLOBAL EXPOSURE"=2049680, "FIRST TRIGGER BEHAVIOR"=2049696, "CHANNEL SYNC"=1852352, "READOUT DIRECTION"=4211904, "PRE HSYNC COUNT"=1852704] ("Parameter")
                n344 = event-data() -> ("NewVal"=w781:dbl)  [unwired: 1 in, 2 out]
                n345 = call <userlib>:"tm_setparameter_a.vi"("error in (no error)"=w782, "Value in"=w781, "Parameter"=w775, "Handle in"=w780) -> ("error out"=w779:errorcluster, "Handle out"=w778:u32)  [unwired: 6 in]
                n346 = call <userlib>:"tm_getparameter_a.vi"("error in (no error)"=w779, "Parameter"=w775, "Handle in"=w778) -> ("error out"=w776:errorcluster, "Value out"=w774:dbl, "Handle out"=w777:u32)  [unwired: 6 in]
                n347 = local write "EXP"(w774) -> ()
              }
              event "Internal Line Interval": Value Change {
                w788 = u32 4191424 items=["SENSOR MODE"=4212128, "CCD MODE"=4212384, "READOUT MODE"=4211872, "ACTIVE VIEW INDEX"=4343136, "BITS PER CHANNEL"=4342976, "IMAGE PIXEL TYPE"=4343296, "BINNING"=4215968, "EXPOSURE TIME"=2049184, "CONTRAST GAIN"=3163312, "CONTRAST OFFSET"=3163328, "LIGHT MODE"=2114720, "SENSITIVITY"=2114992, "PHOTON IMAGING MODE"=2115200, "HIGH DYNAMIC RANGE MODE"=3163360, "WHITE BALANCE"=3163568, "TEMPERATURE"=2115232, "TEMPERATURE TARGET"=2115264, "SENSOR COOLER FAN"=2115296, "LINEBUNDLE HEIGHT"=4212192, "MECHANICAL SHUTTER"=2115488, "BACK FOCUS POSITION"=8422304, "TRIGGER CONNECTOR"=1066432, "TRIGGER SOURCE"=1066144, "OUTPUT TRIGGER SOURCE"=1852576, "TRIGGER GLOBAL EXPOSURE"=2049680, "FIRST TRIGGER BEHAVIOR"=2049696, "CHANNEL SYNC"=1852352, "READOUT DIRECTION"=4211904, "PRE HSYNC COUNT"=1852704, "INTERNAL LINE SPEED"=4191408, "INTERNAL LINE INVERVAL"=4191424] ("Parameter")
                n348 = event-data() -> ("NewVal"=w792:dbl)  [unwired: 1 in, 2 out]
                n349 = call <userlib>:"tm_setparameter_a.vi"("error in (no error)"=w789, "Value in"=w792, "Parameter"=w788, "Handle in"=w793) -> ("error out"=w790:errorcluster, "Handle out"=w791:u32)  [unwired: 6 in]
                n350 = call <userlib>:"tm_getparameter_a.vi"("error in (no error)"=w790, "Parameter"=w788, "Handle in"=w791) -> ("error out"=w795:errorcluster, "Value out"=w794:dbl, "Handle out"=w796:u32)  [unwired: 6 in]
                n351 = local write "Internal Line Interval"(w794) -> ()
              }
              event "Trigger Source": Value Change {
                w809 = u32 1066144 items=["SENSOR MODE"=4212128, "CCD MODE"=4212384, "READOUT MODE"=4211872, "ACTIVE VIEW INDEX"=4343136, "BITS PER CHANNEL"=4342976, "IMAGE PIXEL TYPE"=4343296, "BINNING"=4215968, "EXPOSURE TIME"=2049184, "CONTRAST GAIN"=3163312, "CONTRAST OFFSET"=3163328, "LIGHT MODE"=2114720, "SENSITIVITY"=2114992, "PHOTON IMAGING MODE"=2115200, "HIGH DYNAMIC RANGE MODE"=3163360, "WHITE BALANCE"=3163568, "TEMPERATURE"=2115232, "TEMPERATURE TARGET"=2115264, "SENSOR COOLER FAN"=2115296, "LINEBUNDLE HEIGHT"=4212192, "MECHANICAL SHUTTER"=2115488, "BACK FOCUS POSITION"=8422304, "TRIGGER CONNECTOR"=1066432, "TRIGGER SOURCE"=1066144, "OUTPUT TRIGGER SOURCE"=1852576, "TRIGGER GLOBAL EXPOSURE"=2049680, "FIRST TRIGGER BEHAVIOR"=2049696, "CHANNEL SYNC"=1852352, "READOUT DIRECTION"=4211904, "PRE HSYNC COUNT"=1852704] ("Parameter")
                n352 = event-data() -> ("NewVal"=w802:sgl)  [unwired: 1 in, 3 out]
                n353 = call <userlib>:"tm_setparameter_a.vi"("error in (no error)"=w808, "Value in"=w802, "Parameter"=w809, "Handle in"=w807) -> ("error out"=w806:errorcluster, "Handle out"=w805:u32)  [unwired: 6 in]
                n354 = call <userlib>:"tm_getparameter_a.vi"("error in (no error)"=w806, "Parameter"=w809, "Handle in"=w805) -> ("error out"=w803:errorcluster, "Handle out"=w804:u32)  [unwired: 6 in, 1 out]
              }
              event "Trigger Mode": Value Change {
                w821 = 1 items=["Snap", "Sequence"] ("Capture mode")
                n355 = event-data() -> ("NewVal"=w815:sgl)  [unwired: 1 in, 4 out]
                n356 = call <userlib>:"tm_stopcapture.vi"("error in (no error)"=w825, "Handle in"=w826) -> ("error out"=w828:errorcluster, "Handle out"=w827:u32)  [unwired: 8 in]
                n357 = call <userlib>:"tm_unpreparecapture.vi"("error in (no error)"=w828, "Handle in"=w827) -> ("error out"=w824:errorcluster, "Handle out"=w823:u32)  [unwired: 8 in]
                n358 = call <userlib>:"tm_setpropertyvalue.vi"("error in (no error)"=w824, "Value in"=w815, "Property ID"=u32 1049104, "Handle in"=w823) -> ("error out"=w819:errorcluster, "Handle out"=w822:u32)  [unwired: 6 in]
                n359 = call <userlib>:"tm_preparecapture.vi"("Capture mode"=w821, "Handle in"=w822) -> ("Buffer Info"=w820:T9, "Handle out"=w818:u32)  [unwired: 6 in, 2 out]
                n360 = call <userlib>:"tm_startcapture_b.vi"("error in (no error)"=w819, "Handle in"=w818) -> ("error out"=w816:errorcluster, "Handle out"=w817:u32)  [unwired: 8 in]
              }
              event "Readout Direction": Value Change {
                w842 = 1 items=["Snap", "Sequence"] ("Capture mode")
                w835 = u32 4211904 items=["SENSOR MODE"=4212128, "CCD MODE"=4212384, "READOUT MODE"=4211872, "ACTIVE VIEW INDEX"=4343136, "BITS PER CHANNEL"=4342976, "IMAGE PIXEL TYPE"=4343296, "BINNING"=4215968, "EXPOSURE TIME"=2049184, "CONTRAST GAIN"=3163312, "CONTRAST OFFSET"=3163328, "LIGHT MODE"=2114720, "SENSITIVITY"=2114992, "PHOTON IMAGING MODE"=2115200, "HIGH DYNAMIC RANGE MODE"=3163360, "WHITE BALANCE"=3163568, "TEMPERATURE"=2115232, "TEMPERATURE TARGET"=2115264, "SENSOR COOLER FAN"=2115296, "LINEBUNDLE HEIGHT"=4212192, "MECHANICAL SHUTTER"=2115488, "BACK FOCUS POSITION"=8422304, "TRIGGER CONNECTOR"=1066432, "TRIGGER SOURCE"=1066144, "OUTPUT TRIGGER SOURCE"=1852576, "TRIGGER GLOBAL EXPOSURE"=2049680, "FIRST TRIGGER BEHAVIOR"=2049696, "CHANNEL SYNC"=1852352, "READOUT DIRECTION"=4211904, "PRE HSYNC COUNT"=1852704] ("Parameter")
                n361 = event-data() -> ("NewVal"=w834:sgl)  [unwired: 1 in, 3 out]
                n362 = call <userlib>:"tm_stopcapture.vi"("error in (no error)"=w847, "Handle in"=w844) -> ("error out"=w848:errorcluster, "Handle out"=w843:u32)  [unwired: 8 in]
                n363 = call <userlib>:"tm_unpreparecapture.vi"("error in (no error)"=w848, "Handle in"=w843) -> ("error out"=w846:errorcluster, "Handle out"=w845:u32)  [unwired: 8 in]
                n364 = call <userlib>:"tm_setparameter_a.vi"("error in (no error)"=w846, "Value in"=w834, "Parameter"=w835, "Handle in"=w845) -> ("error out"=w839:errorcluster, "Handle out"=w838:u32)  [unwired: 6 in]
                n365 = call <userlib>:"tm_preparecapture.vi"("error in (no error)"=w839, "Capture mode"=w842, "Handle in"=w838) -> ("error out"=w840:errorcluster, "Handle out"=w841:u32)  [unwired: 5 in, 2 out]
                n366 = call <userlib>:"tm_startcapture_b.vi"("error in (no error)"=w840, "Handle in"=w841) -> ("error out"=w836:errorcluster, "Handle out"=w837:u32)  [unwired: 8 in]
              }
              event "Camera Readout Mode", "Slit Width / Lines": Value Change {
                w859 = 1 items=["Snap", "Sequence"] ("Capture mode")
                n367 = event-data() -> ()  [unwired: 1 in, 4 out]
                n368 = call <userlib>:"tm_stopcapture.vi"("error in (no error)"=w865, "Handle in"=w866) -> ("error out"=w867:errorcluster, "Handle out"=w863:u32)  [unwired: 8 in]
                n369 = call <userlib>:"tm_unpreparecapture.vi"("error in (no error)"=w867, "Handle in"=w863) -> ("error out"=w858:errorcluster, "Handle out"=w864:u32)  [unwired: 8 in]
                n370 = call <userlib>:"tm_setpropertyvalue.vi"("error in (no error)"=w858, "Value in"="Camera Readout Mode", "Property ID"=u32 4194832, "Handle in"=w864) -> ("error out"=w868:errorcluster, "Handle out"=w869:u32)  [unwired: 6 in]
                n371 = case shown="12" "Camera Readout Mode" {
                  tunnel: w869 -> [w880 w887]
                  tunnel: [w879 w882] -> w862
                  tunnel: w868 -> [w877 w892]
                  tunnel: [w876 w892] -> w860
                  frame 1, Default {
                    n372 = local read "Exposure"() -> (w878:dbl)
                    n373 = call <userlib>:"tm_setpropertyvalue.vi"("error in (no error)"=w877, "Value in"=w878, "Property ID"=u32 2031888, "Handle in"=w880) -> ("error out"=w876:errorcluster, "Handle out"=w879:u32)  [unwired: 6 in]
                  }
                  frame 12 {
                    n374 = local read "Exposure"() -> (w891:dbl)
                    n375 = local read "SVW"() -> (w889:i32)
                    n376 = formula code="slitExpos=frameInter*LW/(LinesToReadout\n+10+LW);\nlineInter = slitExpos / LW;"("frameInter"=w891, "LW"="Slit Width / Lines", "LinesToReadout"=w889) -> ("slitExpos"=w883:dbl, "lineInter"=w886:dbl)
                    n377 = call <userlib>:"tm_setpropertyvalue.vi"("Value in"=w886, "Property ID"=u32 4208720, "Handle in"=w887) -> ("Handle out"=w885:u32)  [unwired: 7 in, 1 out]
                    n378 = call <userlib>:"tm_setpropertyvalue.vi"("Value in"=w883, "Property ID"=u32 2031888, "Handle in"=w885) -> ("Handle out"=w882:u32)  [unwired: 7 in, 1 out]
                  }
                }
                n379 = call <userlib>:"tm_preparecapture.vi"("error in (no error)"=w860, "Capture mode"=w859, "Handle in"=w862) -> ("error out"=w855:errorcluster, "Buffer Info"=w861:T9, "Handle out"=w857:u32)  [unwired: 5 in, 1 out]
                n380 = call <userlib>:"tm_startcapture_b.vi"("error in (no error)"=w855, "Handle in"=w857) -> ("error out"=w854:errorcluster, "Handle out"=w856:u32)  [unwired: 8 in]
              }
              event "Ram Record": Value Change {
                n381 = event-data() -> ()  [unwired: 1 in, 5 out]
                n382 = case shown="True" "Ram Record" {
                  tunnel: w906 -> [w910 w933]
                  tunnel: w905 -> [w909 w930]
                  tunnel: [w910 w916] -> w904
                  tunnel: [w909 w918] -> w903
                  tunnel: [w908 w917] -> w899
                  tunnel: w898 -> [w908 _]
                  tunnel: w896 -> [_ w921]
                  tunnel: [_ w919] -> w895
                  tunnel: w894 -> [_ w915]
                  tunnel: w893 -> [_ w911]
                  frame False {
                  }
                  frame True {
                    w927 = 0 items=["Snap", "Sequence"] ("Capture mode")
                    # "Max 2500"
                    n383 = Flush Queue(queue=w921) -> (queue out=w920:refnum<queue>)  [unwired: 1 in, 2 out]
                    n384 = call <userlib>:"tm_stopcapture.vi"("error in (no error)"=w933, "Handle in"=w930) -> ("error out"=w932:errorcluster, "Handle out"=w931:u32)  [unwired: 8 in]
                    n385 = Bundle By Name(cluster=w911, "State"=Stack_Track."Start Sequence", "Stack Number"=0, "Image"=w915) -> (w912:T4)
                    n386 = call <userlib>:"tm_unpreparecapture.vi"("error in (no error)"=w932, "Handle in"=w931) -> ("error out"=w928:errorcluster, "Handle out"=w929:u32)  [unwired: 8 in]
                    n387 = call <userlib>:"tm_preparecapture.vi"("error in (no error)"=w928, "Frames"="Frames", "Capture mode"=w927, "Handle in"=w929) -> ("error out"=w926:errorcluster, "Buffer Info"=w924:T9, "Handle out"=w925:u32)  [unwired: 4 in, 1 out]
                    n388 = Enqueue Element(queue=w920, element=w912) -> (queue out=w922:refnum<queue>)  [unwired: 2 in, 2 out]
                    n389 = case shown="No Error" w926 {
                      selector: w926 -> [w958 w979]
                      tunnel: w925 -> [w957 w980]
                      tunnel: "Frames" -> [w953 _]
                      tunnel: [w938 w976] -> w918
                      tunnel: w924 -> [w954 _]
                      tunnel: [w937 w978] -> w916
                      tunnel: w922 -> [w952 w974]
                      tunnel: w911 -> [w951 _]
                      tunnel: [w936 w974] -> _
                      tunnel: [FALSE ("value") w988] -> w919
                      tunnel: [w935 w977] -> w917
                      frame No Error {
                        w943 = 1 items=["Snap", "Sequence"] ("Capture mode")
                        # "Frames in RAM"
                        n390 = call <userlib>:"tm_startcapture_b.vi"("error in (no error)"=w958, "Handle in"=w957) -> ("error out"=w955:errorcluster, "Handle out"=w956:u32)  [unwired: 8 in]
                        n391 = for {
                          N: w953 -> [_]
                          tunnel: w956 -> [w973]
                          tunnel: w955 -> [w972]
                          tunnel: w954 -> [w969]
                          tunnel: [w968] -> w949
                          tunnel: [w967] -> w948
                          tunnel: w952 -> [w965]
                          tunnel: Stack_Track."Collecting" ("Enum") -> [w963]
                          tunnel: w951 -> [w961]
                          tunnel: [w960] -> w942
                          i -> [w962]
                          n392 = call <userlib>:"tm_waitnextframe.vi"("error in (no error)"=w972, "Handle in"=w973) -> ("error out"=w970:errorcluster, "Frame Index"=→"Frame Index":i32, "Handle out"=w971:u32)  [unwired: 6 in, 1 out]
                          n393 = call <userlib>:"tm_getframe_a.vi"("error in (no error)"=w970, "Frame Index"=w962, "Buffer Info"=w969, "Handle in"=w971) -> ("error out"=w967:errorcluster, "Data 16"=w959:u16[][], "Handle out"=w968:u32)  [unwired: 3 in, 2 out]
                          n394 = Bundle By Name(cluster=w961, "State"=w963, "Stack Number"=w962, "Image"=w959) -> (w964:T4)
                          n395 = Enqueue Element(queue=w965, element=w964) -> (queue out=w960:refnum<queue>)  [unwired: 2 in, 2 out]
                        }
                        n396 = call <userlib>:"tm_stopcapture.vi"("error in (no error)"=w948, "Handle in"=w949) -> ("error out"=w946:errorcluster, "Handle out"=w947:u32)  [unwired: 8 in]
                        n397 = call <userlib>:"tm_unpreparecapture.vi"("error in (no error)"=w946, "Handle in"=w947) -> ("error out"=w945:errorcluster, "Handle out"=w944:u32)  [unwired: 8 in]
                        n398 = Enqueue Element(queue=w942, element=T4 {"State"=enum."End", "Stack Number"=0, "Image"=[], "Stacks"=0} ("input cluster")) -> (queue out=w936:refnum<queue>)  [unwired: 2 in, 2 out]
                        n399 = call <userlib>:"tm_preparecapture.vi"("error in (no error)"=w945, "Capture mode"=w943, "Handle in"=w944) -> ("error out"=w940:errorcluster, "Buffer Info"=w935:T9, "Handle out"=w939:u32)  [unwired: 5 in, 1 out]
                        n400 = call <userlib>:"tm_startcapture_b.vi"("error in (no error)"=w940, "Handle in"=w939) -> ("error out"=w937:errorcluster, "Handle out"=w938:u32)  [unwired: 8 in]
                      }
                      frame Error {
                        w983 = 1 items=["Snap", "Sequence"] ("Capture mode")
                        # "Prepare camera failure, likely too many frames in stack"
                        n401 = One Button Dialog(message="Too many frames in stack", button name ("OK")="OK") -> (true=w988:bool)
                        n402 = call <userlib>:"tm_stopcapture.vi"("error in (no error)"=w979, "Handle in"=w980) -> ("error out"=w986:errorcluster, "Handle out"=w987:u32)  [unwired: 8 in]
                        n403 = call <userlib>:"tm_unpreparecapture.vi"("error in (no error)"=w986, "Handle in"=w987) -> ("error out"=w985:errorcluster, "Handle out"=w984:u32)  [unwired: 8 in]
                        n404 = Enqueue Element(queue=w974, element=T4 {"State"=enum."Idle", "Stack Number"=0, "Image"=[], "Stacks"=0} ("input cluster")) -> ()  [unwired: 2 in, 3 out]
                        n405 = call <userlib>:"tm_preparecapture.vi"("error in (no error)"=w985, "Capture mode"=w983, "Handle in"=w984) -> ("error out"=w982:errorcluster, "Buffer Info"=w977:T9, "Handle out"=w981:u32)  [unwired: 5 in, 1 out]
                        n406 = call <userlib>:"tm_startcapture_b.vi"("error in (no error)"=w982, "Handle in"=w981) -> ("error out"=w978:errorcluster, "Handle out"=w976:u32)  [unwired: 8 in]
                      }
                    }
                  }
                }
              }
              event "HardDisk Record": Value Change {
                n407 = event-data() -> ()  [unwired: 1 in, 5 out]
                n408 = case shown="True" "HardDisk Record" {
                  tunnel: w1003 -> [w1006 w1022]
                  tunnel: w1002 -> [w1005 w1019]
                  tunnel: [w1006 w1009] -> w1001
                  tunnel: [w1005 w1011] -> w1000
                  tunnel: [w1004 w1010] -> w996
                  tunnel: w995 -> [w1004 _]
                  tunnel: w993 -> [_ w1007]
                  tunnel: [_ w1012] -> w992
                  frame False {
                  }
                  frame True {
                    w1016 = 0 items=["Snap", "Sequence"] ("Capture mode")
                    # "Max 50"
                    n409 = call <userlib>:"tm_stopcapture.vi"("error in (no error)"=w1022, "Handle in"=w1019) -> ("error out"=w1021:errorcluster, "Handle out"=w1020:u32)  [unwired: 8 in]
                    n410 = call <userlib>:"tm_unpreparecapture.vi"("error in (no error)"=w1021, "Handle in"=w1020) -> ("error out"=w1017:errorcluster, "Handle out"=w1018:u32)  [unwired: 8 in]
                    n411 = call <userlib>:"tm_preparecapture.vi"("error in (no error)"=w1017, "Frames"="Frames", "Capture mode"=w1016, "Handle in"=w1018) -> ("error out"=w1015:errorcluster, "Buffer Info"=w1013:T9, "Handle out"=w1014:u32)  [unwired: 4 in, 1 out]
                    n412 = case shown="No Error" w1015 {
                      selector: w1015 -> [w1047 w1060]
                      tunnel: w1014 -> [w1033 w1061]
                      tunnel: [w1036 w1057] -> w1011
                      tunnel: w1013 -> [w1044 _]
                      tunnel: [w1035 w1059] -> w1009
                      tunnel: [FALSE ("value") w1069] -> w1012
                      tunnel: [w1034 w1058] -> w1010
                      tunnel: "Frames" -> [w1030 _]
                      tunnel: w1007 -> [w1024 w1055]
                      frame No Error {
                        w1039 = 1 items=["Snap", "Sequence"] ("Capture mode")
                        n413 = call <userlib>:"tm_startrecorder.vi"("frames"=w1030, "File"="Temp", "Handle in"=w1033) -> ("Handle out"=w1032:u32)  [unwired: 7 in, 1 out]
                        n414 = call <userlib>:"tm_startcapture_b.vi"("error in (no error)"=w1047, "Handle in"=w1032) -> ("error out"=w1045:errorcluster, "Handle out"=w1046:u32)  [unwired: 8 in]
                        n415 = while {
                          tunnel: w1046 -> [w1053]
                          tunnel: w1045 -> [w1052]
                          tunnel: w1044 -> [_]
                          tunnel: [w1054] -> w1042
                          tunnel: w1030 -> [w1049]
                          stop <- w1050 stop-if-true
                          n416 = Wait (ms)(milliseconds to wait=u32 50) -> ()  [unwired: 1 out]
                          n417 = call <userlib>:"tm_getrecorderstatus.vi"("error in (no error)"=w1052, "Handle"=w1053) -> ("error out"=w1054:errorcluster, "Count"=w1048:i32)  [unwired: 6 in, 2 out]
                          n418 = Equal?(x=w1048, y=w1049) -> (x = y?=w1050:bool)
                        }
                        n419 = call <userlib>:"tm_stopcapture.vi"("error in (no error)"=w1042) -> ("error out"=w1029:errorcluster, "Handle out"=w1028:u32)  [unwired: 9 in]
                        n420 = call <userlib>:"tm_stoprecorder.vi"("error in (no error)"=w1029, "Handle in"=w1028) -> ("error out"=w1026:errorcluster, "Handle out"=w1027:u32)  [unwired: 8 in]
                        n421 = Enqueue Element(queue=w1024, element=T4 {"State"=enum."Read Disk", "Stack Number"=0, "Image"=[], "Stacks"=0}, error in (no error)=w1026) -> (error out=w1025:errorcluster)  [unwired: 1 in, 2 out]
                        n422 = call <userlib>:"tm_unpreparecapture.vi"("error in (no error)"=w1025, "Handle in"=w1027) -> ("error out"=w1041:errorcluster, "Handle out"=w1040:u32)  [unwired: 8 in]
                        n423 = call <userlib>:"tm_preparecapture.vi"("error in (no error)"=w1041, "Capture mode"=w1039, "Handle in"=w1040) -> ("error out"=w1038:errorcluster, "Buffer Info"=w1034:T9, "Handle out"=w1037:u32)  [unwired: 5 in, 1 out]
                        n424 = call <userlib>:"tm_startcapture_b.vi"("error in (no error)"=w1038, "Handle in"=w1037) -> ("error out"=w1035:errorcluster, "Handle out"=w1036:u32)  [unwired: 8 in]
                      }
                      frame Error {
                        w1064 = 1 items=["Snap", "Sequence"] ("Capture mode")
                        # "Prepare camera failure, likely too many frames in stack"
                        n425 = One Button Dialog(message="Too many frames in stack", button name ("OK")="OK") -> (true=w1069:bool)
                        n426 = call <userlib>:"tm_stopcapture.vi"("error in (no error)"=w1060, "Handle in"=w1061) -> ("error out"=w1067:errorcluster, "Handle out"=w1068:u32)  [unwired: 8 in]
                        n427 = call <userlib>:"tm_unpreparecapture.vi"("error in (no error)"=w1067, "Handle in"=w1068) -> ("error out"=w1066:errorcluster, "Handle out"=w1065:u32)  [unwired: 8 in]
                        n428 = Enqueue Element(queue=w1055, element=T4 {"State"=enum."STOP", "Stack Number"=0, "Image"=[], "Stacks"=0} ("input cluster")) -> ()  [unwired: 2 in, 3 out]
                        n429 = call <userlib>:"tm_preparecapture.vi"("error in (no error)"=w1066, "Capture mode"=w1064, "Handle in"=w1065) -> ("error out"=w1063:errorcluster, "Buffer Info"=w1058:T9, "Handle out"=w1062:u32)  [unwired: 5 in, 1 out]
                        n430 = call <userlib>:"tm_startcapture_b.vi"("error in (no error)"=w1063, "Handle in"=w1062) -> ("error out"=w1059:errorcluster, "Handle out"=w1057:u32)  [unwired: 8 in]
                      }
                    }
                  }
                }
              }
              event "Scan Mode": Value Change {
                w1072 = u32 4211872 items=["SENSOR MODE"=4212128, "CCD MODE"=4212384, "READOUT MODE"=4211872, "ACTIVE VIEW INDEX"=4343136, "BITS PER CHANNEL"=4342976, "IMAGE PIXEL TYPE"=4343296, "BINNING"=4215968, "EXPOSURE TIME"=2049184, "CONTRAST GAIN"=3163312, "CONTRAST OFFSET"=3163328, "LIGHT MODE"=2114720, "SENSITIVITY"=2114992, "PHOTON IMAGING MODE"=2115200, "HIGH DYNAMIC RANGE MODE"=3163360, "WHITE BALANCE"=3163568, "TEMPERATURE"=2115232, "TEMPERATURE TARGET"=2115264, "SENSOR COOLER FAN"=2115296, "LINEBUNDLE HEIGHT"=4212192, "MECHANICAL SHUTTER"=2115488, "BACK FOCUS POSITION"=8422304, "TRIGGER CONNECTOR"=1066432, "TRIGGER SOURCE"=1066144, "OUTPUT TRIGGER SOURCE"=1852576, "TRIGGER GLOBAL EXPOSURE"=2049680, "FIRST TRIGGER BEHAVIOR"=2049696, "CHANNEL SYNC"=1852352, "READOUT DIRECTION"=4211904, "PRE HSYNC COUNT"=1852704] ("Parameter")
                w1087 = 1 items=["Snap", "Sequence"] ("Capture mode")
                n431 = event-data() -> ("NewVal"=w1077:dbl)  [unwired: 1 in, 2 out]
                n432 = call <userlib>:"tm_stopcapture.vi"("error in (no error)"=w1088, "Handle in"=w1089) -> ("error out"=w1090:errorcluster, "Handle out"=w1091:u32)  [unwired: 8 in]
                n433 = call <userlib>:"tm_unpreparecapture.vi"("error in (no error)"=w1090, "Handle in"=w1091) -> ("error out"=w1075:errorcluster, "Handle out"=w1076:u32)  [unwired: 8 in]
                n434 = call <userlib>:"tm_setparameter_a.vi"("error in (no error)"=w1075, "Value in"=w1077, "Parameter"=w1072, "Handle in"=w1076) -> ("error out"=w1074:errorcluster, "Handle out"=w1073:u32)  [unwired: 6 in]
                n435 = call <userlib>:"tm_getparameter_a.vi"("error in (no error)"=w1074, "Parameter"=w1072, "Handle in"=w1073) -> ("error out"=w1080:errorcluster, "Value out"=w1079:dbl, "Handle out"=w1078:u32)  [unwired: 6 in]
                n436 = local write "SMD"(w1079) -> ()
                n437 = call <userlib>:"tm_preparecapture.vi"("error in (no error)"=w1080, "Capture mode"=w1087, "Handle in"=w1078) -> ("error out"=w1085:errorcluster, "Buffer Info"=w1082:T9, "Handle out"=w1086:u32)  [unwired: 5 in, 1 out]
                n438 = call <userlib>:"tm_startcapture_b.vi"("error in (no error)"=w1085, "Handle in"=w1086) -> ("error out"=w1084:errorcluster, "Handle out"=w1083:u32)  [unwired: 8 in]
              }
              event "Binning": Value Change {
                w1096 = u32 4215968 items=["BINNING"=4215968, "BITS PER CHANNEL"=2, "ACTIVE VIEW INDEX"=3, "CCD MODE"=4, "SENSOR MODE"=5, "READOUT MODE"=6, "EXPOSURE TIME"=7, "CONTRAST GAIN"=8, "CONTRAST OFFSET"=9, "LIGHT MODE"=10, "SENSITIVITY"=11, "WHITE BALANCE"=12, "PHOTON IMAGING MODE"=13, "HIGH DYNAMIC RANGE MODE"=14, "TRIGGER SOURCE"=15, "TRIGGER ACTIVE"=16, "TRIGGER MODE"=17, "TRIGGER POLARITY"=18, "TRIGGER GLOBAL EXPOSURE"=19, "FIRST TRIGGER BEHAVIOR"=20, "TRIGGER TIMES"=21, "OUTPUT TRIGGER POLARITY"=22, "OUTPUT TRIGGER DELAY"=23, "OUTPUT TRIGGER PERIOD"=24, "TEMPERATURE"=25, "TEMPERATURE TARGET"=26, "SENSOR COOLER FAN"=27, "MECHANICAL SHUTTER"=28, "BACK FOCUS POSITION"=29, "FRAMEBUNDLE MODE"=30, "FRAMEBUNDLE NUMBER"=31, "LINEBUNDLE HEIGHT"=32, "TRIGGER CONNECTOR"=33, "IMAGE PIXEL TYPE"=34, "OUTPUT TRIGGER KIND"=35, "READOUT DIRECTION"=36, "CHANNEL SYNC"=37] ("Parameter")
                w1135 = 1 items=["Snap", "Sequence"] ("Capture mode")
                n439 = event-data() -> ("NewVal"=w1097:u16)  [unwired: 1 in, 2 out]
                n440 = call <userlib>:"tm_stopcapture.vi"("error in (no error)"=w1104, "Handle in"=w1105) -> ("error out"=w1102:errorcluster, "Handle out"=w1103:u32)  [unwired: 8 in]
                n441 = call <userlib>:"tm_unpreparecapture.vi"("error in (no error)"=w1102, "Handle in"=w1103) -> ("error out"=w1098:errorcluster, "Handle out"=w1095:u32)  [unwired: 8 in]
                n442 = call <userlib>:"tm_setparameter_a.vi"("error in (no error)"=w1098, "Value in"=w1097, "Parameter"=w1096, "Handle in"=w1095) -> ("error out"=w1099:errorcluster, "Handle out"=w1100:u32)  [unwired: 6 in]
                n443 = call <userlib>:"tm_getarea_a.vi"("error in (no error)"=w1099, "Handle in"=w1100) -> ("error out"=w1123:errorcluster, "V Offset"=w1125:T8, "H Offset"=w1124:T8, "Handle out"=w1122:u32, "H Width"=w1126:T8, "V Width"=w1127:T8)  [unwired: 4 in]
                n444 = Unbundle By Name(w1124) -> ("Value"=w1118:i32, "Minimum"=w1121:i32, "Maximum"=w1120:i32, "Increment"=w1119:i32)
                n445 = Unbundle By Name(w1125) -> ("Value"=w1108:i32, "Minimum"=w1117:i32, "Maximum"=w1116:i32, "Increment"=w1115:i32)
                n446 = Unbundle By Name(w1126) -> ("Value"=w1107:i32, "Minimum"=w1114:i32, "Maximum"=w1113:i32, "Increment"=w1112:i32)
                n447 = Unbundle By Name(w1127) -> ("Value"=w1106:i32, "Minimum"=w1111:i32, "Maximum"=w1110:i32, "Increment"=w1109:i32)
                n448 = property on="H Offset" class="DigNum (strict)"("Value"=w1118, "Minimum"=w1121, "Maximum"=w1120, "Increment"=w1119) -> ()  [unwired: 2 in, 2 out]
                n449 = property on="V Offset" class="DigNum (strict)"("Value"=w1108, "Minimum"=w1117, "Maximum"=w1116, "Increment"=w1115) -> ()  [unwired: 2 in, 2 out]
                n450 = property on="H Width" class="DigNum (strict)"("Value"=w1107, "Minimum"=w1114, "Maximum"=w1113, "Increment"=w1112) -> ()  [unwired: 2 in, 2 out]
                n451 = property on="V Width" class="DigNum (strict)"("Value"=w1106, "Minimum"=w1111, "Maximum"=w1110, "Increment"=w1109) -> ()  [unwired: 2 in, 2 out]
                n452 = local write "SHO"(w1118) -> ()
                n453 = local write "SVO"(w1108) -> ()
                n454 = local write "SHW"(w1107) -> ()
                n455 = local write "SVW"(w1106) -> ()
                n456 = call <userlib>:"tm_preparecapture.vi"("error in (no error)"=w1123, "Capture mode"=w1135, "Handle in"=w1122) -> ("error out"=w1133:errorcluster, "Buffer Info"=w1130:T9, "Handle out"=w1134:u32)  [unwired: 5 in, 1 out]
                n457 = call <userlib>:"tm_startcapture_b.vi"("error in (no error)"=w1133, "Handle in"=w1134) -> ("error out"=w1132:errorcluster, "Handle out"=w1131:u32)  [unwired: 8 in]
              }
              event "H Offset", "H Width", "V Offset", "V Width": Value Change {
                w1180 = 1 items=["Snap", "Sequence"] ("Capture mode")
                n458 = event-data() -> ()  [unwired: 1 in, 4 out]
                n459 = call <userlib>:"tm_stopcapture.vi"("error in (no error)"=w1142, "Handle in"=w1143) -> ("error out"=w1140:errorcluster, "Handle out"=w1141:u32)  [unwired: 8 in]
                n460 = local read "H Offset"() -> (w1146:i32)
                n461 = local read "H Width"() -> (w1147:i32)
                n462 = local read "V Offset"() -> (w1148:i32)
                n463 = local read "V Width"() -> (w1145:i32)
                n464 = call <userlib>:"tm_unpreparecapture.vi"("error in (no error)"=w1140, "Handle in"=w1141) -> ("error out"=w1138:errorcluster, "Handle out"=w1139:u32)  [unwired: 8 in]
                n465 = Bundle("H Offset"=w1146, "V Offset"=w1148, "H Width"=w1147, "V Width"=w1145) -> (w1144:T10)  [unwired: 1 in]
                n466 = call <userlib>:"tm_setarea.vi"("error in (no error)"=w1138, "Sub Region"=w1144, "Handle in"=w1139) -> ("error out"=w1149:errorcluster, "Handle out"=w1150:u32)  [unwired: 7 in]
                n467 = call <userlib>:"tm_getarea_a.vi"("error in (no error)"=w1149, "Handle in"=w1150) -> ("error out"=w1168:errorcluster, "V Offset"=w1170:T8, "H Offset"=w1169:T8, "Handle out"=w1167:u32, "H Width"=w1171:T8, "V Width"=w1172:T8)  [unwired: 4 in]
                n468 = Unbundle By Name(w1169) -> ("Value"=w1163:i32, "Minimum"=w1166:i32, "Maximum"=w1165:i32, "Increment"=w1164:i32)
                n469 = Unbundle By Name(w1170) -> ("Value"=w1153:i32, "Minimum"=w1162:i32, "Maximum"=w1161:i32, "Increment"=w1160:i32)
                n470 = Unbundle By Name(w1171) -> ("Value"=w1152:i32, "Minimum"=w1159:i32, "Maximum"=w1158:i32, "Increment"=w1157:i32)
                n471 = Unbundle By Name(w1172) -> ("Value"=w1151:i32, "Minimum"=w1156:i32, "Maximum"=w1155:i32, "Increment"=w1154:i32)
                n472 = property on="H Offset" class="DigNum (strict)"("Value"=w1163, "Minimum"=w1166, "Maximum"=w1165, "Increment"=w1164) -> ()  [unwired: 2 in, 2 out]
                n473 = property on="V Offset" class="DigNum (strict)"("Value"=w1153, "Minimum"=w1162, "Maximum"=w1161, "Increment"=w1160) -> ()  [unwired: 2 in, 2 out]
                n474 = property on="H Width" class="DigNum (strict)"("Value"=w1152, "Minimum"=w1159, "Maximum"=w1158, "Increment"=w1157) -> ()  [unwired: 2 in, 2 out]
                n475 = property on="V Width" class="DigNum (strict)"("Value"=w1151, "Minimum"=w1156, "Maximum"=w1155, "Increment"=w1154) -> ()  [unwired: 2 in, 2 out]
                n476 = local write "SHO"(w1163) -> ()
                n477 = local write "SVO"(w1153) -> ()
                n478 = local write "SHW"(w1152) -> ()
                n479 = local write "SVW"(w1151) -> ()
                n480 = call <userlib>:"tm_preparecapture.vi"("error in (no error)"=w1168, "Capture mode"=w1180, "Handle in"=w1167) -> ("error out"=w1178:errorcluster, "Buffer Info"=w1175:T9, "Handle out"=w1179:u32)  [unwired: 5 in, 1 out]
                n481 = call <userlib>:"tm_startcapture_b.vi"("error in (no error)"=w1178, "Handle in"=w1179) -> ("error out"=w1177:errorcluster, "Handle out"=w1176:u32)  [unwired: 8 in]
              }
            }
            n482 = local read "stop"() -> (w684:bool)
            n483 = Unbundle By Name(w693) -> ("status"=w706:bool)
            n484 = Compound Arithmetic op=OR(w706, w684, w688) -> (w705:bool)
          }
        }
        frame Enabled {
        }
      }
      n485 = call <userlib>:"tm_stopcapture.vi"("error in (no error)"=w26, "Handle in"=w27) -> ("error out"=w73:errorcluster, "Handle out"=w74:u32)  [unwired: 8 in]
      n486 = call <userlib>:"tm_unpreparecapture.vi"("error in (no error)"=w73, "Handle in"=w74) -> ("error out"=w72:errorcluster, "Handle out"=w75:u32)  [unwired: 8 in]
      n487 = call <userlib>:"tm_closecamera.vi"("error in (no error)"=w72, "Handle in"=w75) -> ("error out"=w100:errorcluster)  [unwired: 9 in]
      n488 = call <userlib>:"tm_deinitialize.vi"("error in (no error)"=w100) -> ("error out"=w22:errorcluster)  [unwired: 10 in]
      n489 = Release Queue(queue=w21, error in (no error)=w22) -> (error out=w20:errorcluster)  [unwired: 1 in, 2 out]
      n490 = Release Queue(queue=w18, error in (no error)=w20) -> (error out=w19:errorcluster)  [unwired: 1 in, 2 out]
    }
  }
  "error out" <- w3
